vi "longterm_testV2.vi"() -> ()   [LabVIEW 2017]
uses:
  <vilib>/Math Plots/2D Math Plots/2D Error Bar/2D Error Bar XCtrl/2D Error Bar.xctl
  <vilib>/Math Plots/2D Math Plots/2D Error Bar/2D Error Bar Datatype/2D Error Bar Datatype.lvclass
  <vilib>/Math Plots/2D Math Plots/2D Error Bar/2D Error Bar Datatype/Public/Plot Helper (Fixed).vi
panel:
  out "Vcc":T1(graph)=[{"seconds since 1Jan1904"=timestamp(3822506942.315674 s since 1904-01-01), "mean[ps]"=986.572265625}, {"seconds since 1Jan1904"=timestamp(3822507243.6711025 s since 1904-01-01), "mean[ps]"=973.388671875}, {"seconds since 1Jan1904"=timestamp(3822507545.1626496 s since 1904-01-01), "mean[ps]"=984.375}, {"seconds since 1Jan1904"=timestamp(3822507846.553396 s since 1904-01-01), "mean[ps]"=972.65625}, {"seconds since 1Jan1904"=timestamp(3822508148.061275 s since 1904-01-01), "mean[ps]"=972.65625}, {"seconds since 1Jan1904"=timestamp(3822508449.501727 s since 1904-01-01), "mean[ps]"=974.12109375}, {"seconds since 1Jan1904"=timestamp(3822508750.8988624 s since 1904-01-01), "mean[ps]"=974.12109375}, {"seconds since 1Jan1904"=timestamp(3822509052.3161006 s since 1904-01-01), "mean[ps]"=984.375}, {"seconds since 1Jan1904"=timestamp(3822509353.734636 s since 1904-01-01), "mean[ps]"=986.572265625}, {"seconds since 1Jan1904"=timestamp(3822509655.1987686 s since 1904-01-01), "mean[ps]"=972.65625}, {"seconds since 1Jan1904"=timestamp(3822509956.4995074 s since 1904-01-01), "mean[ps]"=974.12109375}, {"seconds since 1Jan1904"=timestamp(3822510257.982245 s since 1904-01-01), "mean[ps]"=984.375}, {"seconds since 1Jan1904"=timestamp(3822510559.3960705 s since 1904-01-01), "mean[ps]"=984.375}, {"seconds since 1Jan1904"=timestamp(3822510860.7242055 s since 1904-01-01), "mean[ps]"=985.83984375}, {"seconds since 1Jan1904"=timestamp(3822511162.215253 s since 1904-01-01), "mean[ps]"=973.388671875}, {"seconds since 1Jan1904"=timestamp(3822511463.639548 s since 1904-01-01), "mean[ps]"=983.642578125}, {"seconds since 1Jan1904"=timestamp(3822511765.766084 s since 1904-01-01), "mean[ps]"=995.361328125}, {"seconds since 1Jan1904"=timestamp(3822512067.2562017 s since 1904-01-01), "mean[ps]"=984.375}, {"seconds since 1Jan1904"=timestamp(3822512368.655607 s since 1904-01-01), "mean[ps]"=995.361328125}, {"seconds since 1Jan1904"=timestamp(3822512670.1464553 s since 1904-01-01), "mean[ps]"=995.361328125}, {"seconds since 1Jan1904"=timestamp(3822512971.507803 s since 1904-01-01), "mean[ps]"=974.12109375}, {"seconds since 1Jan1904"=timestamp(3822513272.925895 s since 1904-01-01), "mean[ps]"=985.107421875}, {"seconds since 1Jan1904"=timestamp(3822513574.303528 s since 1904-01-01), "mean[ps]"=995.361328125}, {"seconds since 1Jan1904"=timestamp(3822513875.706833 s since 1904-01-01), "mean[ps]"=984.375}, {"seconds since 1Jan1904"=timestamp(3822514177.255216 s since 1904-01-01), "mean[ps]"=994.62890625}, {"seconds since 1Jan1904"=timestamp(3822514478.6136312 s since 1904-01-01), "mean[ps]"=984.375}, {"seconds since 1Jan1904"=timestamp(3822514780.1012654 s since 1904-01-01), "mean[ps]"=983.642578125}, {"seconds since 1Jan1904"=timestamp(3822515081.6113095 s since 1904-01-01), "mean[ps]"=985.83984375}, {"seconds since 1Jan1904"=timestamp(3822515382.9461207 s since 1904-01-01), "mean[ps]"=983.642578125}, {"seconds since 1Jan1904"=timestamp(3822515684.3828025 s since 1904-01-01), "mean[ps]"=986.572265625}, {"seconds since 1Jan1904"=timestamp(3822515985.8758097 s since 1904-01-01), "mean[ps]"=995.361328125}, {"seconds since 1Jan1904"=timestamp(3822516287.3353777 s since 1904-01-01), "mean[ps]"=972.65625}, {"seconds since 1Jan1904"=timestamp(3822516588.8038144 s since 1904-01-01), "mean[ps]"=972.65625}, {"seconds since 1Jan1904"=timestamp(3822516890.2282143 s since 1904-01-01), "mean[ps]"=973.388671875}, {"seconds since 1Jan1904"=timestamp(3822517191.6262407 s since 1904-01-01), "mean[ps]"=985.83984375}, {"seconds since 1Jan1904"=timestamp(3822517493.0924606 s since 1904-01-01), "mean[ps]"=972.65625}, {"seconds since 1Jan1904"=timestamp(3822517794.532418 s since 1904-01-01), "mean[ps]"=994.62890625}, {"seconds since 1Jan1904"=timestamp(3822518095.958946 s since 1904-01-01), "mean[ps]"=986.572265625}, {"seconds since 1Jan1904"=timestamp(3822518397.3720393 s since 1904-01-01), "mean[ps]"=994.62890625}, {"seconds since 1Jan1904"=timestamp(3822518698.777503 s since 1904-01-01), "mean[ps]"=987.3046875}, {"seconds since 1Jan1904"=timestamp(3822519000.1937714 s since 1904-01-01), "mean[ps]"=984.375}, {"seconds since 1Jan1904"=timestamp(3822519301.6194086 s since 1904-01-01), "mean[ps]"=974.12109375}, {"seconds since 1Jan1904"=timestamp(3822519603.042124 s since 1904-01-01), "mean[ps]"=973.388671875}, {"seconds since 1Jan1904"=timestamp(3822519904.578883 s since 1904-01-01), "mean[ps]"=984.375}, {"seconds since 1Jan1904"=timestamp(3822520206.0544343 s since 1904-01-01), "mean[ps]"=986.572265625}, {"seconds since 1Jan1904"=timestamp(3822520507.509728 s since 1904-01-01), "mean[ps]"=985.83984375}, {"seconds since 1Jan1904"=timestamp(3822520809.0371656 s since 1904-01-01), "mean[ps]"=976.318359375}, {"seconds since 1Jan1904"=timestamp(3822521110.5518007 s since 1904-01-01), "mean[ps]"=981.4453125}, {"seconds since 1Jan1904"=timestamp(3822521411.9820223 s since 1904-01-01), "mean[ps]"=974.12109375}, {"seconds since 1Jan1904"=timestamp(3822521713.4490914 s since 1904-01-01), "mean[ps]"=972.65625}, {"seconds since 1Jan1904"=timestamp(3822522014.93792 s since 1904-01-01), "mean[ps]"=995.361328125}, {"seconds since 1Jan1904"=timestamp(3822522316.3927464 s since 1904-01-01), "mean[ps]"=984.375}, {"seconds since 1Jan1904"=timestamp(3822522617.8067694 s since 1904-01-01), "mean[ps]"=985.107421875}, {"seconds since 1Jan1904"=timestamp(3822522919.2539024 s since 1904-01-01), "mean[ps]"=984.375}, {"seconds since 1Jan1904"=timestamp(3822523220.6865177 s since 1904-01-01), "mean[ps]"=974.12109375}, {"seconds since 1Jan1904"=timestamp(3822523522.1590304 s since 1904-01-01), "mean[ps]"=985.83984375}, {"seconds since 1Jan1904"=timestamp(3822523823.5384583 s since 1904-01-01), "mean[ps]"=985.107421875}, {"seconds since 1Jan1904"=timestamp(3822524124.9813824 s since 1904-01-01), "mean[ps]"=973.388671875}, {"seconds since 1Jan1904"=timestamp(3822524426.491788 s since 1904-01-01), "mean[ps]"=972.65625}, {"seconds since 1Jan1904"=timestamp(3822524727.9125314 s since 1904-01-01), "mean[ps]"=974.853515625}, {"seconds since 1Jan1904"=timestamp(3822525029.379265 s since 1904-01-01), "mean[ps]"=994.62890625}, {"seconds since 1Jan1904"=timestamp(3822525330.781236 s since 1904-01-01), "mean[ps]"=995.361328125}, {"seconds since 1Jan1904"=timestamp(3822525632.329557 s since 1904-01-01), "mean[ps]"=982.177734375}, {"seconds since 1Jan1904"=timestamp(3822525933.784519 s since 1904-01-01), "mean[ps]"=994.62890625}, {"seconds since 1Jan1904"=timestamp(3822526235.2852225 s since 1904-01-01), "mean[ps]"=974.12109375}, {"seconds since 1Jan1904"=timestamp(3822526536.779774 s since 1904-01-01), "mean[ps]"=985.83984375}, {"seconds since 1Jan1904"=timestamp(3822526838.2156734 s since 1904-01-01), "mean[ps]"=985.107421875}, {"seconds since 1Jan1904"=timestamp(3822527139.721087 s since 1904-01-01), "mean[ps]"=994.62890625}, {"seconds since 1Jan1904"=timestamp(3822527441.1896977 s since 1904-01-01), "mean[ps]"=985.107421875}, {"seconds since 1Jan1904"=timestamp(3822527742.6183696 s since 1904-01-01), "mean[ps]"=972.65625}, {"seconds since 1Jan1904"=timestamp(3822528044.0890102 s since 1904-01-01), "mean[ps]"=985.83984375}, {"seconds since 1Jan1904"=timestamp(3822528345.503568 s since 1904-01-01), "mean[ps]"=985.107421875}, {"seconds since 1Jan1904"=timestamp(3822528646.8947263 s since 1904-01-01), "mean[ps]"=986.572265625}, {"seconds since 1Jan1904"=timestamp(3822528948.387137 s since 1904-01-01), "mean[ps]"=995.361328125}, {"seconds since 1Jan1904"=timestamp(3822529249.822836 s since 1904-01-01), "mean[ps]"=973.388671875}, {"seconds since 1Jan1904"=timestamp(3822529551.2237015 s since 1904-01-01), "mean[ps]"=982.91015625}, {"seconds since 1Jan1904"=timestamp(3822529852.7132487 s since 1904-01-01), "mean[ps]"=972.65625}, {"seconds since 1Jan1904"=timestamp(3822530154.13355 s since 1904-01-01), "mean[ps]"=986.572265625}, {"seconds since 1Jan1904"=timestamp(3822530455.5063615 s since 1904-01-01), "mean[ps]"=973.388671875}, {"seconds since 1Jan1904"=timestamp(3822530756.906737 s since 1904-01-01), "mean[ps]"=972.65625}, {"seconds since 1Jan1904"=timestamp(3822531058.404439 s since 1904-01-01), "mean[ps]"=993.896484375}, {"seconds since 1Jan1904"=timestamp(3822531359.808485 s since 1904-01-01), "mean[ps]"=982.177734375}, {"seconds since 1Jan1904"=timestamp(3822531661.336039 s since 1904-01-01), "mean[ps]"=975.5859375}, {"seconds since 1Jan1904"=timestamp(3822531962.7850113 s since 1904-01-01), "mean[ps]"=984.375}, {"seconds since 1Jan1904"=timestamp(3822532264.2264094 s since 1904-01-01), "mean[ps]"=973.388671875}, {"seconds since 1Jan1904"=timestamp(3822532565.644325 s since 1904-01-01), "mean[ps]"=973.388671875}, {"seconds since 1Jan1904"=timestamp(3822532867.095218 s since 1904-01-01), "mean[ps]"=987.3046875}, {"seconds since 1Jan1904"=timestamp(3822533168.4954033 s since 1904-01-01), "mean[ps]"=982.91015625}, {"seconds since 1Jan1904"=timestamp(3822533470.0292826 s since 1904-01-01), "mean[ps]"=984.375}, {"seconds since 1Jan1904"=timestamp(3822533771.460639 s since 1904-01-01), "mean[ps]"=974.12109375}, {"seconds since 1Jan1904"=timestamp(3822534072.903432 s since 1904-01-01), "mean[ps]"=984.375}, {"seconds since 1Jan1904"=timestamp(3822534374.327941 s since 1904-01-01), "mean[ps]"=985.107421875}, {"seconds since 1Jan1904"=timestamp(3822534675.8510175 s since 1904-01-01), "mean[ps]"=983.642578125}, {"seconds since 1Jan1904"=timestamp(3822534977.3926754 s since 1904-01-01), "mean[ps]"=975.5859375}, {"seconds since 1Jan1904"=timestamp(3822535278.8113256 s since 1904-01-01), "mean[ps]"=985.83984375}, {"seconds since 1Jan1904"=timestamp(3822535580.052392 s since 1904-01-01), "mean[ps]"=973.388671875}, {"seconds since 1Jan1904"=timestamp(3822535881.6109457 s since 1904-01-01), "mean[ps]"=993.1640625}, {"seconds since 1Jan1904"=timestamp(3822536183.1016607 s since 1904-01-01), "mean[ps]"=987.3046875}, {"seconds since 1Jan1904"=timestamp(3822536484.4703193 s since 1904-01-01), "mean[ps]"=994.62890625}, {"seconds since 1Jan1904"=timestamp(3822536786.003652 s since 1904-01-01), "mean[ps]"=993.896484375}, {"seconds since 1Jan1904"=timestamp(3822537087.3877025 s since 1904-01-01), "mean[ps]"=995.361328125}, {"seconds since 1Jan1904"=timestamp(3822537388.9627695 s since 1904-01-01), "mean[ps]"=974.853515625}, {"seconds since 1Jan1904"=timestamp(3822537690.32478 s since 1904-01-01), "mean[ps]"=993.896484375}, {"seconds since 1Jan1904"=timestamp(3822537991.8736057 s since 1904-01-01), "mean[ps]"=994.62890625}, {"seconds since 1Jan1904"=timestamp(3822538293.281887 s since 1904-01-01), "mean[ps]"=972.65625}, {"seconds since 1Jan1904"=timestamp(3822538594.700456 s since 1904-01-01), "mean[ps]"=972.65625}, {"seconds since 1Jan1904"=timestamp(3822538896.2253175 s since 1904-01-01), "mean[ps]"=972.65625}, {"seconds since 1Jan1904"=timestamp(3822539197.7020054 s since 1904-01-01), "mean[ps]"=985.83984375}, {"seconds since 1Jan1904"=timestamp(3822539499.1529503 s since 1904-01-01), "mean[ps]"=995.361328125}, {"seconds since 1Jan1904"=timestamp(3822539800.5176826 s since 1904-01-01), "mean[ps]"=983.642578125}, {"seconds since 1Jan1904"=timestamp(3822540101.955672 s since 1904-01-01), "mean[ps]"=972.65625}, {"seconds since 1Jan1904"=timestamp(3822540403.389026 s since 1904-01-01), "mean[ps]"=985.83984375}, {"seconds since 1Jan1904"=timestamp(3822540704.8647823 s since 1904-01-01), "mean[ps]"=986.572265625}, {"seconds since 1Jan1904"=timestamp(3822541006.2905207 s since 1904-01-01), "mean[ps]"=985.83984375}, {"seconds since 1Jan1904"=timestamp(3822541307.8066297 s since 1904-01-01), "mean[ps]"=986.572265625}, {"seconds since 1Jan1904"=timestamp(3822541609.3079934 s since 1904-01-01), "mean[ps]"=972.65625}, {"seconds since 1Jan1904"=timestamp(3822541910.788964 s since 1904-01-01), "mean[ps]"=985.107421875}, {"seconds since 1Jan1904"=timestamp(3822542212.360313 s since 1904-01-01), "mean[ps]"=984.375}, {"seconds since 1Jan1904"=timestamp(3822542513.8452806 s since 1904-01-01), "mean[ps]"=984.375}, {"seconds since 1Jan1904"=timestamp(3822542815.328869 s since 1904-01-01), "mean[ps]"=972.65625}, {"seconds since 1Jan1904"=timestamp(3822543116.8031616 s since 1904-01-01), "mean[ps]"=982.91015625}, {"seconds since 1Jan1904"=timestamp(3822543418.253579 s since 1904-01-01), "mean[ps]"=985.83984375}, {"seconds since 1Jan1904"=timestamp(3822543719.8005633 s since 1904-01-01), "mean[ps]"=982.91015625}, {"seconds since 1Jan1904"=timestamp(3822544021.284577 s since 1904-01-01), "mean[ps]"=982.177734375}, {"seconds since 1Jan1904"=timestamp(3822544322.8030105 s since 1904-01-01), "mean[ps]"=986.572265625}, {"seconds since 1Jan1904"=timestamp(3822544624.2975945 s since 1904-01-01), "mean[ps]"=984.375}, {"seconds since 1Jan1904"=timestamp(3822544925.818383 s since 1904-01-01), "mean[ps]"=985.107421875}, {"seconds since 1Jan1904"=timestamp(3822545227.2305446 s since 1904-01-01), "mean[ps]"=983.642578125}, {"seconds since 1Jan1904"=timestamp(3822545528.6374345 s since 1904-01-01), "mean[ps]"=995.361328125}, {"seconds since 1Jan1904"=timestamp(3822545830.161919 s since 1904-01-01), "mean[ps]"=972.65625}, {"seconds since 1Jan1904"=timestamp(3822546131.6581616 s since 1904-01-01), "mean[ps]"=985.107421875}, {"seconds since 1Jan1904"=timestamp(3822546433.1208367 s since 1904-01-01), "mean[ps]"=973.388671875}, {"seconds since 1Jan1904"=timestamp(3822546734.5235424 s since 1904-01-01), "mean[ps]"=984.375}, {"seconds since 1Jan1904"=timestamp(3822547035.9215217 s since 1904-01-01), "mean[ps]"=972.65625}, {"seconds since 1Jan1904"=timestamp(3822547337.4649706 s since 1904-01-01), "mean[ps]"=972.65625}, {"seconds since 1Jan1904"=timestamp(3822547638.88064 s since 1904-01-01), "mean[ps]"=982.91015625}, {"seconds since 1Jan1904"=timestamp(3822547940.3121905 s since 1904-01-01), "mean[ps]"=973.388671875}, {"seconds since 1Jan1904"=timestamp(3822548241.74978 s since 1904-01-01), "mean[ps]"=984.375}, {"seconds since 1Jan1904"=timestamp(3822548543.2799606 s since 1904-01-01), "mean[ps]"=973.388671875}, {"seconds since 1Jan1904"=timestamp(3822548844.742632 s since 1904-01-01), "mean[ps]"=985.107421875}, {"seconds since 1Jan1904"=timestamp(3822549146.149104 s since 1904-01-01), "mean[ps]"=984.375}, {"seconds since 1Jan1904"=timestamp(3822549447.533661 s since 1904-01-01), "mean[ps]"=985.107421875}, {"seconds since 1Jan1904"=timestamp(3822549748.9579425 s since 1904-01-01), "mean[ps]"=995.361328125}, {"seconds since 1Jan1904"=timestamp(3822550050.4716654 s since 1904-01-01), "mean[ps]"=985.83984375}, {"seconds since 1Jan1904"=timestamp(3822550351.947339 s since 1904-01-01), "mean[ps]"=985.107421875}, {"seconds since 1Jan1904"=timestamp(3822550653.458123 s since 1904-01-01), "mean[ps]"=983.642578125}, {"seconds since 1Jan1904"=timestamp(3822550954.99518 s since 1904-01-01), "mean[ps]"=985.83984375}, {"seconds since 1Jan1904"=timestamp(3822551256.5036974 s since 1904-01-01), "mean[ps]"=985.107421875}, {"seconds since 1Jan1904"=timestamp(3822551558.0137887 s since 1904-01-01), "mean[ps]"=995.361328125}, {"seconds since 1Jan1904"=timestamp(3822551859.5051265 s since 1904-01-01), "mean[ps]"=995.361328125}, {"seconds since 1Jan1904"=timestamp(3822552161.039615 s since 1904-01-01), "mean[ps]"=986.572265625}, {"seconds since 1Jan1904"=timestamp(3822552462.609901 s since 1904-01-01), "mean[ps]"=974.853515625}, {"seconds since 1Jan1904"=timestamp(3822552764.000548 s since 1904-01-01), "mean[ps]"=985.107421875}, {"seconds since 1Jan1904"=timestamp(3822553065.419496 s since 1904-01-01), "mean[ps]"=984.375}, {"seconds since 1Jan1904"=timestamp(3822553366.9214015 s since 1904-01-01), "mean[ps]"=995.361328125}, {"seconds since 1Jan1904"=timestamp(3822553668.2656054 s since 1904-01-01), "mean[ps]"=984.375}, {"seconds since 1Jan1904"=timestamp(3822553969.7844114 s since 1904-01-01), "mean[ps]"=984.375}, {"seconds since 1Jan1904"=timestamp(3822554271.2343993 s since 1904-01-01), "mean[ps]"=984.375}, {"seconds since 1Jan1904"=timestamp(3822554572.7825623 s since 1904-01-01), "mean[ps]"=983.642578125}, {"seconds since 1Jan1904"=timestamp(3822554874.2372446 s since 1904-01-01), "mean[ps]"=984.375}, {"seconds since 1Jan1904"=timestamp(3822555175.792369 s since 1904-01-01), "mean[ps]"=985.107421875}, {"seconds since 1Jan1904"=timestamp(3822555477.2372074 s since 1904-01-01), "mean[ps]"=972.65625}, {"seconds since 1Jan1904"=timestamp(3822555778.701035 s since 1904-01-01), "mean[ps]"=987.3046875}, {"seconds since 1Jan1904"=timestamp(3822556080.2516418 s since 1904-01-01), "mean[ps]"=974.12109375}, {"seconds since 1Jan1904"=timestamp(3822556381.757804 s since 1904-01-01), "mean[ps]"=985.107421875}, {"seconds since 1Jan1904"=timestamp(3822556683.148675 s since 1904-01-01), "mean[ps]"=972.65625}, {"seconds since 1Jan1904"=timestamp(3822556984.6444607 s since 1904-01-01), "mean[ps]"=985.107421875}, {"seconds since 1Jan1904"=timestamp(3822557286.095585 s since 1904-01-01), "mean[ps]"=982.91015625}, {"seconds since 1Jan1904"=timestamp(3822557587.5588975 s since 1904-01-01), "mean[ps]"=985.83984375}, {"seconds since 1Jan1904"=timestamp(3822557889.0395904 s since 1904-01-01), "mean[ps]"=974.853515625}, {"seconds since 1Jan1904"=timestamp(3822558190.4474607 s since 1904-01-01), "mean[ps]"=985.107421875}, {"seconds since 1Jan1904"=timestamp(3822558492.0190606 s since 1904-01-01), "mean[ps]"=983.642578125}, {"seconds since 1Jan1904"=timestamp(3822558793.477814 s since 1904-01-01), "mean[ps]"=985.83984375}, {"seconds since 1Jan1904"=timestamp(3822559094.921321 s since 1904-01-01), "mean[ps]"=994.62890625}, {"seconds since 1Jan1904"=timestamp(3822559396.4460673 s since 1904-01-01), "mean[ps]"=984.375}, {"seconds since 1Jan1904"=timestamp(3822559697.9183455 s since 1904-01-01), "mean[ps]"=973.388671875}, {"seconds since 1Jan1904"=timestamp(3822559999.3983808 s since 1904-01-01), "mean[ps]"=994.62890625}, {"seconds since 1Jan1904"=timestamp(3822560300.8987856 s since 1904-01-01), "mean[ps]"=974.12109375}, {"seconds since 1Jan1904"=timestamp(3822560602.3556256 s since 1904-01-01), "mean[ps]"=974.853515625}, {"seconds since 1Jan1904"=timestamp(3822560903.899011 s since 1904-01-01), "mean[ps]"=981.4453125}, {"seconds since 1Jan1904"=timestamp(3822561205.442392 s since 1904-01-01), "mean[ps]"=994.62890625}, {"seconds since 1Jan1904"=timestamp(3822561506.864459 s since 1904-01-01), "mean[ps]"=986.572265625}, {"seconds since 1Jan1904"=timestamp(3822561808.4265895 s since 1904-01-01), "mean[ps]"=985.107421875}, {"seconds since 1Jan1904"=timestamp(3822562109.9678545 s since 1904-01-01), "mean[ps]"=972.65625}, {"seconds since 1Jan1904"=timestamp(3822562411.5341334 s since 1904-01-01), "mean[ps]"=982.91015625}, {"seconds since 1Jan1904"=timestamp(3822562712.998142 s since 1904-01-01), "mean[ps]"=994.62890625}, {"seconds since 1Jan1904"=timestamp(3822563014.480204 s since 1904-01-01), "mean[ps]"=995.361328125}, {"seconds since 1Jan1904"=timestamp(3822563315.9980226 s since 1904-01-01), "mean[ps]"=973.388671875}, {"seconds since 1Jan1904"=timestamp(3822563617.240683 s since 1904-01-01), "mean[ps]"=972.65625}, {"seconds since 1Jan1904"=timestamp(3822563918.749057 s since 1904-01-01), "mean[ps]"=984.375}, {"seconds since 1Jan1904"=timestamp(3822564220.254855 s since 1904-01-01), "mean[ps]"=985.107421875}, {"seconds since 1Jan1904"=timestamp(3822564521.8313217 s since 1904-01-01), "mean[ps]"=985.83984375}, {"seconds since 1Jan1904"=timestamp(3822564823.2753153 s since 1904-01-01), "mean[ps]"=985.107421875}, {"seconds since 1Jan1904"=timestamp(3822565124.701639 s since 1904-01-01), "mean[ps]"=985.83984375}, {"seconds since 1Jan1904"=timestamp(3822565426.1726537 s since 1904-01-01), "mean[ps]"=986.572265625}, {"seconds since 1Jan1904"=timestamp(3822565727.6830926 s since 1904-01-01), "mean[ps]"=972.65625}, {"seconds since 1Jan1904"=timestamp(3822566029.165819 s since 1904-01-01), "mean[ps]"=974.12109375}, {"seconds since 1Jan1904"=timestamp(3822566330.740963 s since 1904-01-01), "mean[ps]"=972.65625}, {"seconds since 1Jan1904"=timestamp(3822566632.249509 s since 1904-01-01), "mean[ps]"=983.642578125}, {"seconds since 1Jan1904"=timestamp(3822566933.704676 s since 1904-01-01), "mean[ps]"=972.65625}, {"seconds since 1Jan1904"=timestamp(3822567235.209213 s since 1904-01-01), "mean[ps]"=984.375}, {"seconds since 1Jan1904"=timestamp(3822567536.6946225 s since 1904-01-01), "mean[ps]"=994.62890625}, {"seconds since 1Jan1904"=timestamp(3822567838.169631 s since 1904-01-01), "mean[ps]"=982.91015625}, {"seconds since 1Jan1904"=timestamp(3822568139.6286063 s since 1904-01-01), "mean[ps]"=985.83984375}, {"seconds since 1Jan1904"=timestamp(3822568441.096488 s since 1904-01-01), "mean[ps]"=995.361328125}, {"seconds since 1Jan1904"=timestamp(3822568742.5332594 s since 1904-01-01), "mean[ps]"=984.375}, {"seconds since 1Jan1904"=timestamp(3822569044.0896015 s since 1904-01-01), "mean[ps]"=972.65625}, {"seconds since 1Jan1904"=timestamp(3822569345.551961 s since 1904-01-01), "mean[ps]"=987.3046875}, {"seconds since 1Jan1904"=timestamp(3822569647.024821 s since 1904-01-01), "mean[ps]"=994.62890625}, {"seconds since 1Jan1904"=timestamp(3822569948.559713 s since 1904-01-01), "mean[ps]"=986.572265625}, {"seconds since 1Jan1904"=timestamp(3822570249.9499383 s since 1904-01-01), "mean[ps]"=995.361328125}, {"seconds since 1Jan1904"=timestamp(3822570551.4543366 s since 1904-01-01), "mean[ps]"=974.12109375}, {"seconds since 1Jan1904"=timestamp(3822570852.907388 s since 1904-01-01), "mean[ps]"=985.107421875}, {"seconds since 1Jan1904"=timestamp(3822571154.3613434 s since 1904-01-01), "mean[ps]"=973.388671875}, {"seconds since 1Jan1904"=timestamp(3822571455.875889 s since 1904-01-01), "mean[ps]"=975.5859375}, {"seconds since 1Jan1904"=timestamp(3822571757.4035335 s since 1904-01-01), "mean[ps]"=984.375}, {"seconds since 1Jan1904"=timestamp(3822572058.8738127 s since 1904-01-01), "mean[ps]"=983.642578125}, {"seconds since 1Jan1904"=timestamp(3822572360.3478255 s since 1904-01-01), "mean[ps]"=995.361328125}, {"seconds since 1Jan1904"=timestamp(3822572661.834789 s since 1904-01-01), "mean[ps]"=985.107421875}, {"seconds since 1Jan1904"=timestamp(3822572963.3136296 s since 1904-01-01), "mean[ps]"=983.642578125}, {"seconds since 1Jan1904"=timestamp(3822573264.8089194 s since 1904-01-01), "mean[ps]"=987.3046875}, {"seconds since 1Jan1904"=timestamp(3822573566.2905793 s since 1904-01-01), "mean[ps]"=983.642578125}, {"seconds since 1Jan1904"=timestamp(3822573867.753861 s since 1904-01-01), "mean[ps]"=982.91015625}, {"seconds since 1Jan1904"=timestamp(3822574169.3307586 s since 1904-01-01), "mean[ps]"=985.83984375}, {"seconds since 1Jan1904"=timestamp(3822574470.7852354 s since 1904-01-01), "mean[ps]"=988.037109375}, {"seconds since 1Jan1904"=timestamp(3822574772.1922865 s since 1904-01-01), "mean[ps]"=984.375}, {"seconds since 1Jan1904"=timestamp(3822575073.6485744 s since 1904-01-01), "mean[ps]"=982.91015625}, {"seconds since 1Jan1904"=timestamp(3822575375.0628457 s since 1904-01-01), "mean[ps]"=994.62890625}, {"seconds since 1Jan1904"=timestamp(3822575676.540885 s since 1904-01-01), "mean[ps]"=984.375}, {"seconds since 1Jan1904"=timestamp(3822575978.110875 s since 1904-01-01), "mean[ps]"=972.65625}, {"seconds since 1Jan1904"=timestamp(3822576279.6679864 s since 1904-01-01), "mean[ps]"=982.91015625}, {"seconds since 1Jan1904"=timestamp(3822576581.2032743 s since 1904-01-01), "mean[ps]"=984.375}, {"seconds since 1Jan1904"=timestamp(3822576882.6405673 s since 1904-01-01), "mean[ps]"=985.83984375}, {"seconds since 1Jan1904"=timestamp(3822577184.1204553 s since 1904-01-01), "mean[ps]"=994.62890625}, {"seconds since 1Jan1904"=timestamp(3822577485.6404696 s since 1904-01-01), "mean[ps]"=973.388671875}, {"seconds since 1Jan1904"=timestamp(3822577787.095057 s since 1904-01-01), "mean[ps]"=982.91015625}, {"seconds since 1Jan1904"=timestamp(3822578088.553026 s since 1904-01-01), "mean[ps]"=984.375}, {"seconds since 1Jan1904"=timestamp(3822578390.115008 s since 1904-01-01), "mean[ps]"=982.91015625}, {"seconds since 1Jan1904"=timestamp(3822578691.551293 s since 1904-01-01), "mean[ps]"=995.361328125}, {"seconds since 1Jan1904"=timestamp(3822578992.9199705 s since 1904-01-01), "mean[ps]"=994.62890625}, {"seconds since 1Jan1904"=timestamp(3822579294.3933854 s since 1904-01-01), "mean[ps]"=995.361328125}, {"seconds since 1Jan1904"=timestamp(3822579595.918991 s since 1904-01-01), "mean[ps]"=995.361328125}, {"seconds since 1Jan1904"=timestamp(3822579897.4222097 s since 1904-01-01), "mean[ps]"=982.177734375}, {"seconds since 1Jan1904"=timestamp(3822580198.9128265 s since 1904-01-01), "mean[ps]"=975.5859375}, {"seconds since 1Jan1904"=timestamp(3822580500.314174 s since 1904-01-01), "mean[ps]"=986.572265625}, {"seconds since 1Jan1904"=timestamp(3822580801.8501215 s since 1904-01-01), "mean[ps]"=988.037109375}, {"seconds since 1Jan1904"=timestamp(3822581103.3778 s since 1904-01-01), "mean[ps]"=973.388671875}, {"seconds since 1Jan1904"=timestamp(3822581404.880745 s since 1904-01-01), "mean[ps]"=983.642578125}, {"seconds since 1Jan1904"=timestamp(3822581706.4360175 s since 1904-01-01), "mean[ps]"=984.375}, {"seconds since 1Jan1904"=timestamp(3822582007.8203206 s since 1904-01-01), "mean[ps]"=995.361328125}, {"seconds since 1Jan1904"=timestamp(3822582309.2484713 s since 1904-01-01), "mean[ps]"=995.361328125}, {"seconds since 1Jan1904"=timestamp(3822582610.7182074 s since 1904-01-01), "mean[ps]"=974.12109375}, {"seconds since 1Jan1904"=timestamp(3822582912.221481 s since 1904-01-01), "mean[ps]"=980.712890625}, {"seconds since 1Jan1904"=timestamp(3822583213.701206 s since 1904-01-01), "mean[ps]"=973.388671875}, {"seconds since 1Jan1904"=timestamp(3822583515.2400217 s since 1904-01-01), "mean[ps]"=982.177734375}, {"seconds since 1Jan1904"=timestamp(3822583816.7411456 s since 1904-01-01), "mean[ps]"=982.91015625}, {"seconds since 1Jan1904"=timestamp(3822584118.2147617 s since 1904-01-01), "mean[ps]"=982.91015625}, {"seconds since 1Jan1904"=timestamp(3822584419.675927 s since 1904-01-01), "mean[ps]"=995.361328125}, {"seconds since 1Jan1904"=timestamp(3822584721.0923023 s since 1904-01-01), "mean[ps]"=986.572265625}, {"seconds since 1Jan1904"=timestamp(3822585022.5496383 s since 1904-01-01), "mean[ps]"=976.318359375}, {"seconds since 1Jan1904"=timestamp(3822585324.043527 s since 1904-01-01), "mean[ps]"=974.853515625}, {"seconds since 1Jan1904"=timestamp(3822585625.471996 s since 1904-01-01), "mean[ps]"=972.65625}, {"seconds since 1Jan1904"=timestamp(3822585926.8942423 s since 1904-01-01), "mean[ps]"=975.5859375}, {"seconds since 1Jan1904"=timestamp(3822586228.3225694 s since 1904-01-01), "mean[ps]"=986.572265625}, {"seconds since 1Jan1904"=timestamp(3822586529.8338766 s since 1904-01-01), "mean[ps]"=986.572265625}, {"seconds since 1Jan1904"=timestamp(3822586831.2920294 s since 1904-01-01), "mean[ps]"=986.572265625}, {"seconds since 1Jan1904"=timestamp(3822587132.7088814 s since 1904-01-01), "mean[ps]"=985.107421875}, {"seconds since 1Jan1904"=timestamp(3822587434.1071906 s since 1904-01-01), "mean[ps]"=986.572265625}, {"seconds since 1Jan1904"=timestamp(3822587735.3207207 s since 1904-01-01), "mean[ps]"=986.572265625}, {"seconds since 1Jan1904"=timestamp(3822588036.7855854 s since 1904-01-01), "mean[ps]"=985.107421875}, {"seconds since 1Jan1904"=timestamp(3822588338.3446593 s since 1904-01-01), "mean[ps]"=982.91015625}, {"seconds since 1Jan1904"=timestamp(3822588639.839839 s since 1904-01-01), "mean[ps]"=992.431640625}, {"seconds since 1Jan1904"=timestamp(3822588941.288984 s since 1904-01-01), "mean[ps]"=985.83984375}, {"seconds since 1Jan1904"=timestamp(3822589242.7402463 s since 1904-01-01), "mean[ps]"=995.361328125}, {"seconds since 1Jan1904"=timestamp(3822589544.2098656 s since 1904-01-01), "mean[ps]"=983.642578125}, {"seconds since 1Jan1904"=timestamp(3822589845.6971216 s since 1904-01-01), "mean[ps]"=973.388671875}, {"seconds since 1Jan1904"=timestamp(3822590147.2125216 s since 1904-01-01), "mean[ps]"=982.91015625}, {"seconds since 1Jan1904"=timestamp(3822590448.640258 s since 1904-01-01), "mean[ps]"=972.65625}, {"seconds since 1Jan1904"=timestamp(3822590750.1391034 s since 1904-01-01), "mean[ps]"=993.896484375}, {"seconds since 1Jan1904"=timestamp(3822591051.5836415 s since 1904-01-01), "mean[ps]"=976.318359375}, {"seconds since 1Jan1904"=timestamp(3822591352.9831247 s since 1904-01-01), "mean[ps]"=973.388671875}, {"seconds since 1Jan1904"=timestamp(3822591654.485979 s since 1904-01-01), "mean[ps]"=986.572265625}, {"seconds since 1Jan1904"=timestamp(3822591955.859042 s since 1904-01-01), "mean[ps]"=995.361328125}, {"seconds since 1Jan1904"=timestamp(3822592257.408669 s since 1904-01-01), "mean[ps]"=972.65625}, {"seconds since 1Jan1904"=timestamp(3822592558.932187 s since 1904-01-01), "mean[ps]"=984.375}, {"seconds since 1Jan1904"=timestamp(3822592860.391513 s since 1904-01-01), "mean[ps]"=993.896484375}, {"seconds since 1Jan1904"=timestamp(3822593161.860652 s since 1904-01-01), "mean[ps]"=983.642578125}, {"seconds since 1Jan1904"=timestamp(3822593463.385323 s since 1904-01-01), "mean[ps]"=985.107421875}, {"seconds since 1Jan1904"=timestamp(3822593764.8500686 s since 1904-01-01), "mean[ps]"=985.83984375}, {"seconds since 1Jan1904"=timestamp(3822594066.308588 s since 1904-01-01), "mean[ps]"=981.4453125}, {"seconds since 1Jan1904"=timestamp(3822594367.780607 s since 1904-01-01), "mean[ps]"=985.83984375}, {"seconds since 1Jan1904"=timestamp(3822594669.2577024 s since 1904-01-01), "mean[ps]"=982.91015625}, {"seconds since 1Jan1904"=timestamp(3822594970.726291 s since 1904-01-01), "mean[ps]"=985.83984375}, {"seconds since 1Jan1904"=timestamp(3822595272.1390114 s since 1904-01-01), "mean[ps]"=973.388671875}, {"seconds since 1Jan1904"=timestamp(3822595573.6779704 s since 1904-01-01), "mean[ps]"=994.62890625}, {"seconds since 1Jan1904"=timestamp(3822595875.2007656 s since 1904-01-01), "mean[ps]"=984.375}, {"seconds since 1Jan1904"=timestamp(3822596176.6578298 s since 1904-01-01), "mean[ps]"=985.107421875}, {"seconds since 1Jan1904"=timestamp(3822596478.2190976 s since 1904-01-01), "mean[ps]"=974.12109375}, {"seconds since 1Jan1904"=timestamp(3822596779.7422447 s since 1904-01-01), "mean[ps]"=985.107421875}, {"seconds since 1Jan1904"=timestamp(3822597081.1809144 s since 1904-01-01), "mean[ps]"=985.83984375}, {"seconds since 1Jan1904"=timestamp(3822597382.686327 s since 1904-01-01), "mean[ps]"=985.83984375}, {"seconds since 1Jan1904"=timestamp(3822597684.2478952 s since 1904-01-01), "mean[ps]"=984.375}, {"seconds since 1Jan1904"=timestamp(3822597985.7226458 s since 1904-01-01), "mean[ps]"=984.375}, {"seconds since 1Jan1904"=timestamp(3822598287.212348 s since 1904-01-01), "mean[ps]"=995.361328125}, {"seconds since 1Jan1904"=timestamp(3822598588.6026154 s since 1904-01-01), "mean[ps]"=993.896484375}, {"seconds since 1Jan1904"=timestamp(3822598890.0572553 s since 1904-01-01), "mean[ps]"=987.3046875}, {"seconds since 1Jan1904"=timestamp(3822599191.425584 s since 1904-01-01), "mean[ps]"=973.388671875}, {"seconds since 1Jan1904"=timestamp(3822599492.866769 s since 1904-01-01), "mean[ps]"=985.107421875}, {"seconds since 1Jan1904"=timestamp(3822599794.2904983 s since 1904-01-01), "mean[ps]"=973.388671875}, {"seconds since 1Jan1904"=timestamp(3822600095.7871695 s since 1904-01-01), "mean[ps]"=973.388671875}, {"seconds since 1Jan1904"=timestamp(3822600397.4508214 s since 1904-01-01), "mean[ps]"=983.642578125}, {"seconds since 1Jan1904"=timestamp(3822600698.83722 s since 1904-01-01), "mean[ps]"=994.62890625}, {"seconds since 1Jan1904"=timestamp(3822601000.21038 s since 1904-01-01), "mean[ps]"=973.388671875}, {"seconds since 1Jan1904"=timestamp(3822601301.7260976 s since 1904-01-01), "mean[ps]"=973.388671875}]
  in  "mean[ps] 4":dbl=-0.9 format="%0.2f"
  in  "mean[ps] 3":dbl=-0.7 format="%0.2f"
  in  "seconds since 1Jan1904 3":timestamp=timestamp(3822019516.105 s since 1904-01-01)
  in  "mean[ps] 2":dbl=-0.16666666666666666 format="%0.2f"
  in  "seconds since 1Jan1904 2":timestamp=timestamp(3822019276.105 s since 1904-01-01)
  out "Mean 2":T2(graph)=[{[{"seconds since 1Jan1904 2"=timestamp(3822019276.105 s since 1904-01-01), "mean[ps] 2"=-0.16666666666666666}, {"seconds since 1Jan1904 2"=timestamp(3822019516.105 s since 1904-01-01), "mean[ps] 2"=-0.7}]}, {[{"seconds since 1Jan1904 2"=timestamp(3822019276.105 s since 1904-01-01), "mean[ps] 2"=-0.16666666666666666}, {"seconds since 1Jan1904 2"=timestamp(3822019516.105 s since 1904-01-01), "mean[ps] 2"=-0.9}]}]
  out "temperature":T1(graph)=[{"seconds since 1Jan1904"=timestamp(3822506942.315674 s since 1904-01-01), "mean[ps]"=40.85004882812501}, {"seconds since 1Jan1904"=timestamp(3822507243.6711025 s since 1904-01-01), "mean[ps]"=41.465252685546886}, {"seconds since 1Jan1904"=timestamp(3822507545.1626496 s since 1904-01-01), "mean[ps]"=41.465252685546886}, {"seconds since 1Jan1904"=timestamp(3822507846.553396 s since 1904-01-01), "mean[ps]"=40.97308959960941}, {"seconds since 1Jan1904"=timestamp(3822508148.061275 s since 1904-01-01), "mean[ps]"=41.588293457031284}, {"seconds since 1Jan1904"=timestamp(3822508449.501727 s since 1904-01-01), "mean[ps]"=41.342211914062545}, {"seconds since 1Jan1904"=timestamp(3822508750.8988624 s since 1904-01-01), "mean[ps]"=72.47152709960943}, {"seconds since 1Jan1904"=timestamp(3822509052.3161006 s since 1904-01-01), "mean[ps]"=10.335937500000057}, {"seconds since 1Jan1904"=timestamp(3822509353.734636 s since 1904-01-01), "mean[ps]"=41.342211914062545}, {"seconds since 1Jan1904"=timestamp(3822509655.1987686 s since 1904-01-01), "mean[ps]"=40.85004882812501}, {"seconds since 1Jan1904"=timestamp(3822509956.4995074 s since 1904-01-01), "mean[ps]"=41.588293457031284}, {"seconds since 1Jan1904"=timestamp(3822510257.982245 s since 1904-01-01), "mean[ps]"=72.96369018554691}, {"seconds since 1Jan1904"=timestamp(3822510559.3960705 s since 1904-01-01), "mean[ps]"=41.09613037109381}, {"seconds since 1Jan1904"=timestamp(3822510860.7242055 s since 1904-01-01), "mean[ps]"=40.85004882812501}, {"seconds since 1Jan1904"=timestamp(3822511162.215253 s since 1904-01-01), "mean[ps]"=41.21917114257815}, {"seconds since 1Jan1904"=timestamp(3822511463.639548 s since 1904-01-01), "mean[ps]"=42.32653808593756}, {"seconds since 1Jan1904"=timestamp(3822511765.766084 s since 1904-01-01), "mean[ps]"=41.83437500000002}, {"seconds since 1Jan1904"=timestamp(3822512067.2562017 s since 1904-01-01), "mean[ps]"=41.588293457031284}, {"seconds since 1Jan1904"=timestamp(3822512368.655607 s since 1904-01-01), "mean[ps]"=42.32653808593756}, {"seconds since 1Jan1904"=timestamp(3822512670.1464553 s since 1904-01-01), "mean[ps]"=41.71133422851568}, {"seconds since 1Jan1904"=timestamp(3822512971.507803 s since 1904-01-01), "mean[ps]"=10.335937500000057}, {"seconds since 1Jan1904"=timestamp(3822513272.925895 s since 1904-01-01), "mean[ps]"=10.458978271484398}, {"seconds since 1Jan1904"=timestamp(3822513574.303528 s since 1904-01-01), "mean[ps]"=42.20349731445316}, {"seconds since 1Jan1904"=timestamp(3822513875.706833 s since 1904-01-01), "mean[ps]"=73.0867309570313}, {"seconds since 1Jan1904"=timestamp(3822514177.255216 s since 1904-01-01), "mean[ps]"=42.08045654296876}, {"seconds since 1Jan1904"=timestamp(3822514478.6136312 s since 1904-01-01), "mean[ps]"=72.96369018554691}, {"seconds since 1Jan1904"=timestamp(3822514780.1012654 s since 1904-01-01), "mean[ps]"=10.828100585937534}, {"seconds since 1Jan1904"=timestamp(3822515081.6113095 s since 1904-01-01), "mean[ps]"=11.074182128906273}, {"seconds since 1Jan1904"=timestamp(3822515382.9461207 s since 1904-01-01), "mean[ps]"=72.59456787109377}, {"seconds since 1Jan1904"=timestamp(3822515684.3828025 s since 1904-01-01), "mean[ps]"=41.83437500000002}, {"seconds since 1Jan1904"=timestamp(3822515985.8758097 s since 1904-01-01), "mean[ps]"=42.32653808593756}, {"seconds since 1Jan1904"=timestamp(3822516287.3353777 s since 1904-01-01), "mean[ps]"=42.32653808593756}, {"seconds since 1Jan1904"=timestamp(3822516588.8038144 s since 1904-01-01), "mean[ps]"=42.20349731445316}, {"seconds since 1Jan1904"=timestamp(3822516890.2282143 s since 1904-01-01), "mean[ps]"=42.818701171875034}, {"seconds since 1Jan1904"=timestamp(3822517191.6262407 s since 1904-01-01), "mean[ps]"=42.695660400390636}, {"seconds since 1Jan1904"=timestamp(3822517493.0924606 s since 1904-01-01), "mean[ps]"=42.4495788574219}, {"seconds since 1Jan1904"=timestamp(3822517794.532418 s since 1904-01-01), "mean[ps]"=41.95741577148442}, {"seconds since 1Jan1904"=timestamp(3822518095.958946 s since 1904-01-01), "mean[ps]"=43.18782348632817}, {"seconds since 1Jan1904"=timestamp(3822518397.3720393 s since 1904-01-01), "mean[ps]"=42.572619628906295}, {"seconds since 1Jan1904"=timestamp(3822518698.777503 s since 1904-01-01), "mean[ps]"=43.06478271484377}, {"seconds since 1Jan1904"=timestamp(3822519000.1937714 s since 1904-01-01), "mean[ps]"=42.4495788574219}, {"seconds since 1Jan1904"=timestamp(3822519301.6194086 s since 1904-01-01), "mean[ps]"=42.4495788574219}, {"seconds since 1Jan1904"=timestamp(3822519603.042124 s since 1904-01-01), "mean[ps]"=42.695660400390636}, {"seconds since 1Jan1904"=timestamp(3822519904.578883 s since 1904-01-01), "mean[ps]"=42.94174194335943}, {"seconds since 1Jan1904"=timestamp(3822520206.0544343 s since 1904-01-01), "mean[ps]"=42.695660400390636}, {"seconds since 1Jan1904"=timestamp(3822520507.509728 s since 1904-01-01), "mean[ps]"=42.08045654296876}, {"seconds since 1Jan1904"=timestamp(3822520809.0371656 s since 1904-01-01), "mean[ps]"=43.06478271484377}, {"seconds since 1Jan1904"=timestamp(3822521110.5518007 s since 1904-01-01), "mean[ps]"=42.94174194335943}, {"seconds since 1Jan1904"=timestamp(3822521411.9820223 s since 1904-01-01), "mean[ps]"=42.94174194335943}, {"seconds since 1Jan1904"=timestamp(3822521713.4490914 s since 1904-01-01), "mean[ps]"=42.94174194335943}, {"seconds since 1Jan1904"=timestamp(3822522014.93792 s since 1904-01-01), "mean[ps]"=42.4495788574219}, {"seconds since 1Jan1904"=timestamp(3822522316.3927464 s since 1904-01-01), "mean[ps]"=42.695660400390636}, {"seconds since 1Jan1904"=timestamp(3822522617.8067694 s since 1904-01-01), "mean[ps]"=42.695660400390636}, {"seconds since 1Jan1904"=timestamp(3822522919.2539024 s since 1904-01-01), "mean[ps]"=43.31086425781251}, {"seconds since 1Jan1904"=timestamp(3822523220.6865177 s since 1904-01-01), "mean[ps]"=43.06478271484377}, {"seconds since 1Jan1904"=timestamp(3822523522.1590304 s since 1904-01-01), "mean[ps]"=42.818701171875034}, {"seconds since 1Jan1904"=timestamp(3822523823.5384583 s since 1904-01-01), "mean[ps]"=42.20349731445316}, {"seconds since 1Jan1904"=timestamp(3822524124.9813824 s since 1904-01-01), "mean[ps]"=43.18782348632817}, {"seconds since 1Jan1904"=timestamp(3822524426.491788 s since 1904-01-01), "mean[ps]"=42.818701171875034}, {"seconds since 1Jan1904"=timestamp(3822524727.9125314 s since 1904-01-01), "mean[ps]"=42.94174194335943}, {"seconds since 1Jan1904"=timestamp(3822525029.379265 s since 1904-01-01), "mean[ps]"=42.818701171875034}, {"seconds since 1Jan1904"=timestamp(3822525330.781236 s since 1904-01-01), "mean[ps]"=43.55694580078131}, {"seconds since 1Jan1904"=timestamp(3822525632.329557 s since 1904-01-01), "mean[ps]"=43.31086425781251}, {"seconds since 1Jan1904"=timestamp(3822525933.784519 s since 1904-01-01), "mean[ps]"=42.94174194335943}, {"seconds since 1Jan1904"=timestamp(3822526235.2852225 s since 1904-01-01), "mean[ps]"=43.31086425781251}, {"seconds since 1Jan1904"=timestamp(3822526536.779774 s since 1904-01-01), "mean[ps]"=43.55694580078131}, {"seconds since 1Jan1904"=timestamp(3822526838.2156734 s since 1904-01-01), "mean[ps]"=43.43390502929691}, {"seconds since 1Jan1904"=timestamp(3822527139.721087 s since 1904-01-01), "mean[ps]"=43.18782348632817}, {"seconds since 1Jan1904"=timestamp(3822527441.1896977 s since 1904-01-01), "mean[ps]"=43.43390502929691}, {"seconds since 1Jan1904"=timestamp(3822527742.6183696 s since 1904-01-01), "mean[ps]"=43.18782348632817}, {"seconds since 1Jan1904"=timestamp(3822528044.0890102 s since 1904-01-01), "mean[ps]"=42.32653808593756}, {"seconds since 1Jan1904"=timestamp(3822528345.503568 s since 1904-01-01), "mean[ps]"=43.55694580078131}, {"seconds since 1Jan1904"=timestamp(3822528646.8947263 s since 1904-01-01), "mean[ps]"=43.18782348632817}, {"seconds since 1Jan1904"=timestamp(3822528948.387137 s since 1904-01-01), "mean[ps]"=43.55694580078131}, {"seconds since 1Jan1904"=timestamp(3822529249.822836 s since 1904-01-01), "mean[ps]"=43.43390502929691}, {"seconds since 1Jan1904"=timestamp(3822529551.2237015 s since 1904-01-01), "mean[ps]"=42.94174194335943}, {"seconds since 1Jan1904"=timestamp(3822529852.7132487 s since 1904-01-01), "mean[ps]"=43.31086425781251}, {"seconds since 1Jan1904"=timestamp(3822530154.13355 s since 1904-01-01), "mean[ps]"=43.55694580078131}, {"seconds since 1Jan1904"=timestamp(3822530455.5063615 s since 1904-01-01), "mean[ps]"=44.049108886718784}, {"seconds since 1Jan1904"=timestamp(3822530756.906737 s since 1904-01-01), "mean[ps]"=43.926068115234386}, {"seconds since 1Jan1904"=timestamp(3822531058.404439 s since 1904-01-01), "mean[ps]"=43.55694580078131}, {"seconds since 1Jan1904"=timestamp(3822531359.808485 s since 1904-01-01), "mean[ps]"=43.67998657226565}, {"seconds since 1Jan1904"=timestamp(3822531661.336039 s since 1904-01-01), "mean[ps]"=43.31086425781251}, {"seconds since 1Jan1904"=timestamp(3822531962.7850113 s since 1904-01-01), "mean[ps]"=43.06478271484377}, {"seconds since 1Jan1904"=timestamp(3822532264.2264094 s since 1904-01-01), "mean[ps]"=42.08045654296876}, {"seconds since 1Jan1904"=timestamp(3822532565.644325 s since 1904-01-01), "mean[ps]"=43.06478271484377}, {"seconds since 1Jan1904"=timestamp(3822532867.095218 s since 1904-01-01), "mean[ps]"=42.20349731445316}, {"seconds since 1Jan1904"=timestamp(3822533168.4954033 s since 1904-01-01), "mean[ps]"=42.08045654296876}, {"seconds since 1Jan1904"=timestamp(3822533470.0292826 s since 1904-01-01), "mean[ps]"=43.31086425781251}, {"seconds since 1Jan1904"=timestamp(3822533771.460639 s since 1904-01-01), "mean[ps]"=42.818701171875034}, {"seconds since 1Jan1904"=timestamp(3822534072.903432 s since 1904-01-01), "mean[ps]"=42.94174194335943}, {"seconds since 1Jan1904"=timestamp(3822534374.327941 s since 1904-01-01), "mean[ps]"=42.94174194335943}, {"seconds since 1Jan1904"=timestamp(3822534675.8510175 s since 1904-01-01), "mean[ps]"=42.572619628906295}, {"seconds since 1Jan1904"=timestamp(3822534977.3926754 s since 1904-01-01), "mean[ps]"=43.06478271484377}, {"seconds since 1Jan1904"=timestamp(3822535278.8113256 s since 1904-01-01), "mean[ps]"=43.31086425781251}, {"seconds since 1Jan1904"=timestamp(3822535580.052392 s since 1904-01-01), "mean[ps]"=42.695660400390636}, {"seconds since 1Jan1904"=timestamp(3822535881.6109457 s since 1904-01-01), "mean[ps]"=43.31086425781251}, {"seconds since 1Jan1904"=timestamp(3822536183.1016607 s since 1904-01-01), "mean[ps]"=42.08045654296876}, {"seconds since 1Jan1904"=timestamp(3822536484.4703193 s since 1904-01-01), "mean[ps]"=42.695660400390636}, {"seconds since 1Jan1904"=timestamp(3822536786.003652 s since 1904-01-01), "mean[ps]"=42.818701171875034}, {"seconds since 1Jan1904"=timestamp(3822537087.3877025 s since 1904-01-01), "mean[ps]"=42.32653808593756}, {"seconds since 1Jan1904"=timestamp(3822537388.9627695 s since 1904-01-01), "mean[ps]"=42.4495788574219}, {"seconds since 1Jan1904"=timestamp(3822537690.32478 s since 1904-01-01), "mean[ps]"=42.572619628906295}, {"seconds since 1Jan1904"=timestamp(3822537991.8736057 s since 1904-01-01), "mean[ps]"=42.32653808593756}, {"seconds since 1Jan1904"=timestamp(3822538293.281887 s since 1904-01-01), "mean[ps]"=42.818701171875034}, {"seconds since 1Jan1904"=timestamp(3822538594.700456 s since 1904-01-01), "mean[ps]"=42.695660400390636}, {"seconds since 1Jan1904"=timestamp(3822538896.2253175 s since 1904-01-01), "mean[ps]"=43.31086425781251}, {"seconds since 1Jan1904"=timestamp(3822539197.7020054 s since 1904-01-01), "mean[ps]"=42.572619628906295}, {"seconds since 1Jan1904"=timestamp(3822539499.1529503 s since 1904-01-01), "mean[ps]"=42.818701171875034}, {"seconds since 1Jan1904"=timestamp(3822539800.5176826 s since 1904-01-01), "mean[ps]"=42.818701171875034}, {"seconds since 1Jan1904"=timestamp(3822540101.955672 s since 1904-01-01), "mean[ps]"=42.818701171875034}, {"seconds since 1Jan1904"=timestamp(3822540403.389026 s since 1904-01-01), "mean[ps]"=42.08045654296876}, {"seconds since 1Jan1904"=timestamp(3822540704.8647823 s since 1904-01-01), "mean[ps]"=43.31086425781251}, {"seconds since 1Jan1904"=timestamp(3822541006.2905207 s since 1904-01-01), "mean[ps]"=43.43390502929691}, {"seconds since 1Jan1904"=timestamp(3822541307.8066297 s since 1904-01-01), "mean[ps]"=43.06478271484377}, {"seconds since 1Jan1904"=timestamp(3822541609.3079934 s since 1904-01-01), "mean[ps]"=42.94174194335943}, {"seconds since 1Jan1904"=timestamp(3822541910.788964 s since 1904-01-01), "mean[ps]"=42.20349731445316}, {"seconds since 1Jan1904"=timestamp(3822542212.360313 s since 1904-01-01), "mean[ps]"=42.572619628906295}, {"seconds since 1Jan1904"=timestamp(3822542513.8452806 s since 1904-01-01), "mean[ps]"=43.31086425781251}, {"seconds since 1Jan1904"=timestamp(3822542815.328869 s since 1904-01-01), "mean[ps]"=42.4495788574219}, {"seconds since 1Jan1904"=timestamp(3822543116.8031616 s since 1904-01-01), "mean[ps]"=42.08045654296876}, {"seconds since 1Jan1904"=timestamp(3822543418.253579 s since 1904-01-01), "mean[ps]"=10.828100585937534}, {"seconds since 1Jan1904"=timestamp(3822543719.8005633 s since 1904-01-01), "mean[ps]"=43.06478271484377}, {"seconds since 1Jan1904"=timestamp(3822544021.284577 s since 1904-01-01), "mean[ps]"=42.94174194335943}, {"seconds since 1Jan1904"=timestamp(3822544322.8030105 s since 1904-01-01), "mean[ps]"=42.94174194335943}, {"seconds since 1Jan1904"=timestamp(3822544624.2975945 s since 1904-01-01), "mean[ps]"=42.695660400390636}, {"seconds since 1Jan1904"=timestamp(3822544925.818383 s since 1904-01-01), "mean[ps]"=43.06478271484377}, {"seconds since 1Jan1904"=timestamp(3822545227.2305446 s since 1904-01-01), "mean[ps]"=42.818701171875034}, {"seconds since 1Jan1904"=timestamp(3822545528.6374345 s since 1904-01-01), "mean[ps]"=42.695660400390636}, {"seconds since 1Jan1904"=timestamp(3822545830.161919 s since 1904-01-01), "mean[ps]"=42.20349731445316}, {"seconds since 1Jan1904"=timestamp(3822546131.6581616 s since 1904-01-01), "mean[ps]"=43.06478271484377}, {"seconds since 1Jan1904"=timestamp(3822546433.1208367 s since 1904-01-01), "mean[ps]"=42.94174194335943}, {"seconds since 1Jan1904"=timestamp(3822546734.5235424 s since 1904-01-01), "mean[ps]"=42.695660400390636}, {"seconds since 1Jan1904"=timestamp(3822547035.9215217 s since 1904-01-01), "mean[ps]"=42.94174194335943}, {"seconds since 1Jan1904"=timestamp(3822547337.4649706 s since 1904-01-01), "mean[ps]"=43.43390502929691}, {"seconds since 1Jan1904"=timestamp(3822547638.88064 s since 1904-01-01), "mean[ps]"=42.695660400390636}, {"seconds since 1Jan1904"=timestamp(3822547940.3121905 s since 1904-01-01), "mean[ps]"=42.695660400390636}, {"seconds since 1Jan1904"=timestamp(3822548241.74978 s since 1904-01-01), "mean[ps]"=41.95741577148442}, {"seconds since 1Jan1904"=timestamp(3822548543.2799606 s since 1904-01-01), "mean[ps]"=42.818701171875034}, {"seconds since 1Jan1904"=timestamp(3822548844.742632 s since 1904-01-01), "mean[ps]"=42.695660400390636}, {"seconds since 1Jan1904"=timestamp(3822549146.149104 s since 1904-01-01), "mean[ps]"=42.4495788574219}, {"seconds since 1Jan1904"=timestamp(3822549447.533661 s since 1904-01-01), "mean[ps]"=42.4495788574219}, {"seconds since 1Jan1904"=timestamp(3822549748.9579425 s since 1904-01-01), "mean[ps]"=42.695660400390636}, {"seconds since 1Jan1904"=timestamp(3822550050.4716654 s since 1904-01-01), "mean[ps]"=41.95741577148442}, {"seconds since 1Jan1904"=timestamp(3822550351.947339 s since 1904-01-01), "mean[ps]"=42.572619628906295}, {"seconds since 1Jan1904"=timestamp(3822550653.458123 s since 1904-01-01), "mean[ps]"=41.95741577148442}, {"seconds since 1Jan1904"=timestamp(3822550954.99518 s since 1904-01-01), "mean[ps]"=42.572619628906295}, {"seconds since 1Jan1904"=timestamp(3822551256.5036974 s since 1904-01-01), "mean[ps]"=42.818701171875034}, {"seconds since 1Jan1904"=timestamp(3822551558.0137887 s since 1904-01-01), "mean[ps]"=42.4495788574219}, {"seconds since 1Jan1904"=timestamp(3822551859.5051265 s since 1904-01-01), "mean[ps]"=42.695660400390636}, {"seconds since 1Jan1904"=timestamp(3822552161.039615 s since 1904-01-01), "mean[ps]"=42.94174194335943}, {"seconds since 1Jan1904"=timestamp(3822552462.609901 s since 1904-01-01), "mean[ps]"=42.4495788574219}, {"seconds since 1Jan1904"=timestamp(3822552764.000548 s since 1904-01-01), "mean[ps]"=42.4495788574219}, {"seconds since 1Jan1904"=timestamp(3822553065.419496 s since 1904-01-01), "mean[ps]"=42.572619628906295}, {"seconds since 1Jan1904"=timestamp(3822553366.9214015 s since 1904-01-01), "mean[ps]"=43.31086425781251}, {"seconds since 1Jan1904"=timestamp(3822553668.2656054 s since 1904-01-01), "mean[ps]"=42.32653808593756}, {"seconds since 1Jan1904"=timestamp(3822553969.7844114 s since 1904-01-01), "mean[ps]"=42.695660400390636}, {"seconds since 1Jan1904"=timestamp(3822554271.2343993 s since 1904-01-01), "mean[ps]"=42.818701171875034}, {"seconds since 1Jan1904"=timestamp(3822554572.7825623 s since 1904-01-01), "mean[ps]"=42.94174194335943}, {"seconds since 1Jan1904"=timestamp(3822554874.2372446 s since 1904-01-01), "mean[ps]"=43.31086425781251}, {"seconds since 1Jan1904"=timestamp(3822555175.792369 s since 1904-01-01), "mean[ps]"=42.572619628906295}, {"seconds since 1Jan1904"=timestamp(3822555477.2372074 s since 1904-01-01), "mean[ps]"=42.94174194335943}, {"seconds since 1Jan1904"=timestamp(3822555778.701035 s since 1904-01-01), "mean[ps]"=43.43390502929691}, {"seconds since 1Jan1904"=timestamp(3822556080.2516418 s since 1904-01-01), "mean[ps]"=42.4495788574219}, {"seconds since 1Jan1904"=timestamp(3822556381.757804 s since 1904-01-01), "mean[ps]"=42.572619628906295}, {"seconds since 1Jan1904"=timestamp(3822556683.148675 s since 1904-01-01), "mean[ps]"=42.572619628906295}, {"seconds since 1Jan1904"=timestamp(3822556984.6444607 s since 1904-01-01), "mean[ps]"=43.803027343750045}, {"seconds since 1Jan1904"=timestamp(3822557286.095585 s since 1904-01-01), "mean[ps]"=42.32653808593756}, {"seconds since 1Jan1904"=timestamp(3822557587.5588975 s since 1904-01-01), "mean[ps]"=42.695660400390636}, {"seconds since 1Jan1904"=timestamp(3822557889.0395904 s since 1904-01-01), "mean[ps]"=43.06478271484377}, {"seconds since 1Jan1904"=timestamp(3822558190.4474607 s since 1904-01-01), "mean[ps]"=42.94174194335943}, {"seconds since 1Jan1904"=timestamp(3822558492.0190606 s since 1904-01-01), "mean[ps]"=42.94174194335943}, {"seconds since 1Jan1904"=timestamp(3822558793.477814 s since 1904-01-01), "mean[ps]"=42.818701171875034}, {"seconds since 1Jan1904"=timestamp(3822559094.921321 s since 1904-01-01), "mean[ps]"=42.94174194335943}, {"seconds since 1Jan1904"=timestamp(3822559396.4460673 s since 1904-01-01), "mean[ps]"=42.818701171875034}, {"seconds since 1Jan1904"=timestamp(3822559697.9183455 s since 1904-01-01), "mean[ps]"=43.18782348632817}, {"seconds since 1Jan1904"=timestamp(3822559999.3983808 s since 1904-01-01), "mean[ps]"=41.83437500000002}, {"seconds since 1Jan1904"=timestamp(3822560300.8987856 s since 1904-01-01), "mean[ps]"=42.20349731445316}, {"seconds since 1Jan1904"=timestamp(3822560602.3556256 s since 1904-01-01), "mean[ps]"=42.572619628906295}, {"seconds since 1Jan1904"=timestamp(3822560903.899011 s since 1904-01-01), "mean[ps]"=43.06478271484377}, {"seconds since 1Jan1904"=timestamp(3822561205.442392 s since 1904-01-01), "mean[ps]"=42.08045654296876}, {"seconds since 1Jan1904"=timestamp(3822561506.864459 s since 1904-01-01), "mean[ps]"=42.818701171875034}, {"seconds since 1Jan1904"=timestamp(3822561808.4265895 s since 1904-01-01), "mean[ps]"=43.55694580078131}, {"seconds since 1Jan1904"=timestamp(3822562109.9678545 s since 1904-01-01), "mean[ps]"=42.818701171875034}, {"seconds since 1Jan1904"=timestamp(3822562411.5341334 s since 1904-01-01), "mean[ps]"=42.4495788574219}, {"seconds since 1Jan1904"=timestamp(3822562712.998142 s since 1904-01-01), "mean[ps]"=43.43390502929691}, {"seconds since 1Jan1904"=timestamp(3822563014.480204 s since 1904-01-01), "mean[ps]"=43.18782348632817}, {"seconds since 1Jan1904"=timestamp(3822563315.9980226 s since 1904-01-01), "mean[ps]"=41.95741577148442}, {"seconds since 1Jan1904"=timestamp(3822563617.240683 s since 1904-01-01), "mean[ps]"=41.95741577148442}, {"seconds since 1Jan1904"=timestamp(3822563918.749057 s since 1904-01-01), "mean[ps]"=42.818701171875034}, {"seconds since 1Jan1904"=timestamp(3822564220.254855 s since 1904-01-01), "mean[ps]"=42.695660400390636}, {"seconds since 1Jan1904"=timestamp(3822564521.8313217 s since 1904-01-01), "mean[ps]"=42.818701171875034}, {"seconds since 1Jan1904"=timestamp(3822564823.2753153 s since 1904-01-01), "mean[ps]"=42.572619628906295}, {"seconds since 1Jan1904"=timestamp(3822565124.701639 s since 1904-01-01), "mean[ps]"=43.31086425781251}, {"seconds since 1Jan1904"=timestamp(3822565426.1726537 s since 1904-01-01), "mean[ps]"=42.818701171875034}, {"seconds since 1Jan1904"=timestamp(3822565727.6830926 s since 1904-01-01), "mean[ps]"=42.4495788574219}, {"seconds since 1Jan1904"=timestamp(3822566029.165819 s since 1904-01-01), "mean[ps]"=42.695660400390636}, {"seconds since 1Jan1904"=timestamp(3822566330.740963 s since 1904-01-01), "mean[ps]"=42.4495788574219}, {"seconds since 1Jan1904"=timestamp(3822566632.249509 s since 1904-01-01), "mean[ps]"=43.18782348632817}, {"seconds since 1Jan1904"=timestamp(3822566933.704676 s since 1904-01-01), "mean[ps]"=42.572619628906295}, {"seconds since 1Jan1904"=timestamp(3822567235.209213 s since 1904-01-01), "mean[ps]"=42.4495788574219}, {"seconds since 1Jan1904"=timestamp(3822567536.6946225 s since 1904-01-01), "mean[ps]"=42.32653808593756}, {"seconds since 1Jan1904"=timestamp(3822567838.169631 s since 1904-01-01), "mean[ps]"=42.94174194335943}, {"seconds since 1Jan1904"=timestamp(3822568139.6286063 s since 1904-01-01), "mean[ps]"=41.83437500000002}, {"seconds since 1Jan1904"=timestamp(3822568441.096488 s since 1904-01-01), "mean[ps]"=42.32653808593756}, {"seconds since 1Jan1904"=timestamp(3822568742.5332594 s since 1904-01-01), "mean[ps]"=43.06478271484377}, {"seconds since 1Jan1904"=timestamp(3822569044.0896015 s since 1904-01-01), "mean[ps]"=42.94174194335943}, {"seconds since 1Jan1904"=timestamp(3822569345.551961 s since 1904-01-01), "mean[ps]"=42.4495788574219}, {"seconds since 1Jan1904"=timestamp(3822569647.024821 s since 1904-01-01), "mean[ps]"=42.4495788574219}, {"seconds since 1Jan1904"=timestamp(3822569948.559713 s since 1904-01-01), "mean[ps]"=73.20977172851565}, {"seconds since 1Jan1904"=timestamp(3822570249.9499383 s since 1904-01-01), "mean[ps]"=42.4495788574219}, {"seconds since 1Jan1904"=timestamp(3822570551.4543366 s since 1904-01-01), "mean[ps]"=42.32653808593756}, {"seconds since 1Jan1904"=timestamp(3822570852.907388 s since 1904-01-01), "mean[ps]"=42.94174194335943}, {"seconds since 1Jan1904"=timestamp(3822571154.3613434 s since 1904-01-01), "mean[ps]"=42.20349731445316}, {"seconds since 1Jan1904"=timestamp(3822571455.875889 s since 1904-01-01), "mean[ps]"=42.32653808593756}, {"seconds since 1Jan1904"=timestamp(3822571757.4035335 s since 1904-01-01), "mean[ps]"=42.08045654296876}, {"seconds since 1Jan1904"=timestamp(3822572058.8738127 s since 1904-01-01), "mean[ps]"=10.951141357421932}, {"seconds since 1Jan1904"=timestamp(3822572360.3478255 s since 1904-01-01), "mean[ps]"=42.695660400390636}, {"seconds since 1Jan1904"=timestamp(3822572661.834789 s since 1904-01-01), "mean[ps]"=42.572619628906295}, {"seconds since 1Jan1904"=timestamp(3822572963.3136296 s since 1904-01-01), "mean[ps]"=42.695660400390636}, {"seconds since 1Jan1904"=timestamp(3822573264.8089194 s since 1904-01-01), "mean[ps]"=42.08045654296876}, {"seconds since 1Jan1904"=timestamp(3822573566.2905793 s since 1904-01-01), "mean[ps]"=42.08045654296876}, {"seconds since 1Jan1904"=timestamp(3822573867.753861 s since 1904-01-01), "mean[ps]"=42.4495788574219}, {"seconds since 1Jan1904"=timestamp(3822574169.3307586 s since 1904-01-01), "mean[ps]"=73.20977172851565}, {"seconds since 1Jan1904"=timestamp(3822574470.7852354 s since 1904-01-01), "mean[ps]"=43.06478271484377}, {"seconds since 1Jan1904"=timestamp(3822574772.1922865 s since 1904-01-01), "mean[ps]"=42.08045654296876}, {"seconds since 1Jan1904"=timestamp(3822575073.6485744 s since 1904-01-01), "mean[ps]"=41.83437500000002}, {"seconds since 1Jan1904"=timestamp(3822575375.0628457 s since 1904-01-01), "mean[ps]"=42.572619628906295}, {"seconds since 1Jan1904"=timestamp(3822575676.540885 s since 1904-01-01), "mean[ps]"=42.20349731445316}, {"seconds since 1Jan1904"=timestamp(3822575978.110875 s since 1904-01-01), "mean[ps]"=42.695660400390636}, {"seconds since 1Jan1904"=timestamp(3822576279.6679864 s since 1904-01-01), "mean[ps]"=42.32653808593756}, {"seconds since 1Jan1904"=timestamp(3822576581.2032743 s since 1904-01-01), "mean[ps]"=42.32653808593756}, {"seconds since 1Jan1904"=timestamp(3822576882.6405673 s since 1904-01-01), "mean[ps]"=41.83437500000002}, {"seconds since 1Jan1904"=timestamp(3822577184.1204553 s since 1904-01-01), "mean[ps]"=42.32653808593756}, {"seconds since 1Jan1904"=timestamp(3822577485.6404696 s since 1904-01-01), "mean[ps]"=43.06478271484377}, {"seconds since 1Jan1904"=timestamp(3822577787.095057 s since 1904-01-01), "mean[ps]"=42.818701171875034}, {"seconds since 1Jan1904"=timestamp(3822578088.553026 s since 1904-01-01), "mean[ps]"=42.818701171875034}, {"seconds since 1Jan1904"=timestamp(3822578390.115008 s since 1904-01-01), "mean[ps]"=42.4495788574219}, {"seconds since 1Jan1904"=timestamp(3822578691.551293 s since 1904-01-01), "mean[ps]"=42.08045654296876}, {"seconds since 1Jan1904"=timestamp(3822578992.9199705 s since 1904-01-01), "mean[ps]"=42.20349731445316}, {"seconds since 1Jan1904"=timestamp(3822579294.3933854 s since 1904-01-01), "mean[ps]"=41.95741577148442}, {"seconds since 1Jan1904"=timestamp(3822579595.918991 s since 1904-01-01), "mean[ps]"=42.20349731445316}, {"seconds since 1Jan1904"=timestamp(3822579897.4222097 s since 1904-01-01), "mean[ps]"=42.08045654296876}, {"seconds since 1Jan1904"=timestamp(3822580198.9128265 s since 1904-01-01), "mean[ps]"=73.20977172851565}, {"seconds since 1Jan1904"=timestamp(3822580500.314174 s since 1904-01-01), "mean[ps]"=41.83437500000002}, {"seconds since 1Jan1904"=timestamp(3822580801.8501215 s since 1904-01-01), "mean[ps]"=42.695660400390636}, {"seconds since 1Jan1904"=timestamp(3822581103.3778 s since 1904-01-01), "mean[ps]"=42.695660400390636}, {"seconds since 1Jan1904"=timestamp(3822581404.880745 s since 1904-01-01), "mean[ps]"=73.20977172851565}, {"seconds since 1Jan1904"=timestamp(3822581706.4360175 s since 1904-01-01), "mean[ps]"=42.20349731445316}, {"seconds since 1Jan1904"=timestamp(3822582007.8203206 s since 1904-01-01), "mean[ps]"=42.32653808593756}, {"seconds since 1Jan1904"=timestamp(3822582309.2484713 s since 1904-01-01), "mean[ps]"=42.20349731445316}, {"seconds since 1Jan1904"=timestamp(3822582610.7182074 s since 1904-01-01), "mean[ps]"=41.95741577148442}, {"seconds since 1Jan1904"=timestamp(3822582912.221481 s since 1904-01-01), "mean[ps]"=41.588293457031284}, {"seconds since 1Jan1904"=timestamp(3822583213.701206 s since 1904-01-01), "mean[ps]"=42.20349731445316}, {"seconds since 1Jan1904"=timestamp(3822583515.2400217 s since 1904-01-01), "mean[ps]"=10.582019042968795}, {"seconds since 1Jan1904"=timestamp(3822583816.7411456 s since 1904-01-01), "mean[ps]"=42.08045654296876}, {"seconds since 1Jan1904"=timestamp(3822584118.2147617 s since 1904-01-01), "mean[ps]"=41.83437500000002}, {"seconds since 1Jan1904"=timestamp(3822584419.675927 s since 1904-01-01), "mean[ps]"=10.582019042968795}, {"seconds since 1Jan1904"=timestamp(3822584721.0923023 s since 1904-01-01), "mean[ps]"=73.0867309570313}, {"seconds since 1Jan1904"=timestamp(3822585022.5496383 s since 1904-01-01), "mean[ps]"=41.342211914062545}, {"seconds since 1Jan1904"=timestamp(3822585324.043527 s since 1904-01-01), "mean[ps]"=41.83437500000002}, {"seconds since 1Jan1904"=timestamp(3822585625.471996 s since 1904-01-01), "mean[ps]"=42.4495788574219}, {"seconds since 1Jan1904"=timestamp(3822585926.8942423 s since 1904-01-01), "mean[ps]"=73.20977172851565}, {"seconds since 1Jan1904"=timestamp(3822586228.3225694 s since 1904-01-01), "mean[ps]"=41.588293457031284}, {"seconds since 1Jan1904"=timestamp(3822586529.8338766 s since 1904-01-01), "mean[ps]"=10.582019042968795}, {"seconds since 1Jan1904"=timestamp(3822586831.2920294 s since 1904-01-01), "mean[ps]"=41.95741577148442}, {"seconds since 1Jan1904"=timestamp(3822587132.7088814 s since 1904-01-01), "mean[ps]"=41.95741577148442}, {"seconds since 1Jan1904"=timestamp(3822587434.1071906 s since 1904-01-01), "mean[ps]"=42.32653808593756}, {"seconds since 1Jan1904"=timestamp(3822587735.3207207 s since 1904-01-01), "mean[ps]"=73.0867309570313}, {"seconds since 1Jan1904"=timestamp(3822588036.7855854 s since 1904-01-01), "mean[ps]"=42.08045654296876}, {"seconds since 1Jan1904"=timestamp(3822588338.3446593 s since 1904-01-01), "mean[ps]"=72.84064941406251}, {"seconds since 1Jan1904"=timestamp(3822588639.839839 s since 1904-01-01), "mean[ps]"=41.83437500000002}, {"seconds since 1Jan1904"=timestamp(3822588941.288984 s since 1904-01-01), "mean[ps]"=42.20349731445316}, {"seconds since 1Jan1904"=timestamp(3822589242.7402463 s since 1904-01-01), "mean[ps]"=73.0867309570313}, {"seconds since 1Jan1904"=timestamp(3822589544.2098656 s since 1904-01-01), "mean[ps]"=42.08045654296876}, {"seconds since 1Jan1904"=timestamp(3822589845.6971216 s since 1904-01-01), "mean[ps]"=42.32653808593756}, {"seconds since 1Jan1904"=timestamp(3822590147.2125216 s since 1904-01-01), "mean[ps]"=10.828100585937534}, {"seconds since 1Jan1904"=timestamp(3822590448.640258 s since 1904-01-01), "mean[ps]"=10.582019042968795}, {"seconds since 1Jan1904"=timestamp(3822590750.1391034 s since 1904-01-01), "mean[ps]"=10.335937500000057}, {"seconds since 1Jan1904"=timestamp(3822591051.5836415 s since 1904-01-01), "mean[ps]"=41.71133422851568}, {"seconds since 1Jan1904"=timestamp(3822591352.9831247 s since 1904-01-01), "mean[ps]"=42.572619628906295}, {"seconds since 1Jan1904"=timestamp(3822591654.485979 s since 1904-01-01), "mean[ps]"=10.335937500000057}, {"seconds since 1Jan1904"=timestamp(3822591955.859042 s since 1904-01-01), "mean[ps]"=41.95741577148442}, {"seconds since 1Jan1904"=timestamp(3822592257.408669 s since 1904-01-01), "mean[ps]"=73.20977172851565}, {"seconds since 1Jan1904"=timestamp(3822592558.932187 s since 1904-01-01), "mean[ps]"=41.342211914062545}, {"seconds since 1Jan1904"=timestamp(3822592860.391513 s since 1904-01-01), "mean[ps]"=41.83437500000002}, {"seconds since 1Jan1904"=timestamp(3822593161.860652 s since 1904-01-01), "mean[ps]"=41.21917114257815}, {"seconds since 1Jan1904"=timestamp(3822593463.385323 s since 1904-01-01), "mean[ps]"=42.572619628906295}, {"seconds since 1Jan1904"=timestamp(3822593764.8500686 s since 1904-01-01), "mean[ps]"=72.96369018554691}, {"seconds since 1Jan1904"=timestamp(3822594066.308588 s since 1904-01-01), "mean[ps]"=41.21917114257815}, {"seconds since 1Jan1904"=timestamp(3822594367.780607 s since 1904-01-01), "mean[ps]"=10.458978271484398}, {"seconds since 1Jan1904"=timestamp(3822594669.2577024 s since 1904-01-01), "mean[ps]"=42.08045654296876}, {"seconds since 1Jan1904"=timestamp(3822594970.726291 s since 1904-01-01), "mean[ps]"=10.582019042968795}, {"seconds since 1Jan1904"=timestamp(3822595272.1390114 s since 1904-01-01), "mean[ps]"=10.582019042968795}, {"seconds since 1Jan1904"=timestamp(3822595573.6779704 s since 1904-01-01), "mean[ps]"=41.342211914062545}, {"seconds since 1Jan1904"=timestamp(3822595875.2007656 s since 1904-01-01), "mean[ps]"=41.342211914062545}, {"seconds since 1Jan1904"=timestamp(3822596176.6578298 s since 1904-01-01), "mean[ps]"=73.20977172851565}, {"seconds since 1Jan1904"=timestamp(3822596478.2190976 s since 1904-01-01), "mean[ps]"=73.0867309570313}, {"seconds since 1Jan1904"=timestamp(3822596779.7422447 s since 1904-01-01), "mean[ps]"=41.83437500000002}, {"seconds since 1Jan1904"=timestamp(3822597081.1809144 s since 1904-01-01), "mean[ps]"=41.83437500000002}, {"seconds since 1Jan1904"=timestamp(3822597382.686327 s since 1904-01-01), "mean[ps]"=72.84064941406251}, {"seconds since 1Jan1904"=timestamp(3822597684.2478952 s since 1904-01-01), "mean[ps]"=41.71133422851568}, {"seconds since 1Jan1904"=timestamp(3822597985.7226458 s since 1904-01-01), "mean[ps]"=42.20349731445316}, {"seconds since 1Jan1904"=timestamp(3822598287.212348 s since 1904-01-01), "mean[ps]"=10.458978271484398}, {"seconds since 1Jan1904"=timestamp(3822598588.6026154 s since 1904-01-01), "mean[ps]"=41.71133422851568}, {"seconds since 1Jan1904"=timestamp(3822598890.0572553 s since 1904-01-01), "mean[ps]"=42.32653808593756}, {"seconds since 1Jan1904"=timestamp(3822599191.425584 s since 1904-01-01), "mean[ps]"=42.32653808593756}, {"seconds since 1Jan1904"=timestamp(3822599492.866769 s since 1904-01-01), "mean[ps]"=42.818701171875034}, {"seconds since 1Jan1904"=timestamp(3822599794.2904983 s since 1904-01-01), "mean[ps]"=42.695660400390636}, {"seconds since 1Jan1904"=timestamp(3822600095.7871695 s since 1904-01-01), "mean[ps]"=43.18782348632817}, {"seconds since 1Jan1904"=timestamp(3822600397.4508214 s since 1904-01-01), "mean[ps]"=43.67998657226565}, {"seconds since 1Jan1904"=timestamp(3822600698.83722 s since 1904-01-01), "mean[ps]"=43.67998657226565}, {"seconds since 1Jan1904"=timestamp(3822601000.21038 s since 1904-01-01), "mean[ps]"=43.31086425781251}, {"seconds since 1Jan1904"=timestamp(3822601301.7260976 s since 1904-01-01), "mean[ps]"=42.94174194335943}]
  in  "stop":bool
  out "误差线":refnum<class "2D Plot Datatype.lvclass">[](xcontrol)
  out "sigma[ps]":dbl=47.77065519923074 format="%0.2f"
  out "Sigma":T1(graph)=[{"seconds since 1Jan1904"=timestamp(3822506942.315674 s since 1904-01-01), "mean[ps]"=48.159483831069075}, {"seconds since 1Jan1904"=timestamp(3822507243.6711025 s since 1904-01-01), "mean[ps]"=47.408858847112896}, {"seconds since 1Jan1904"=timestamp(3822507545.1626496 s since 1904-01-01), "mean[ps]"=46.61942019456449}, {"seconds since 1Jan1904"=timestamp(3822507846.553396 s since 1904-01-01), "mean[ps]"=48.80667678227107}, {"seconds since 1Jan1904"=timestamp(3822508148.061275 s since 1904-01-01), "mean[ps]"=49.06268181740717}, {"seconds since 1Jan1904"=timestamp(3822508449.501727 s since 1904-01-01), "mean[ps]"=46.182665671236094}, {"seconds since 1Jan1904"=timestamp(3822508750.8988624 s since 1904-01-01), "mean[ps]"=46.257724210817486}, {"seconds since 1Jan1904"=timestamp(3822509052.3161006 s since 1904-01-01), "mean[ps]"=47.361287211332396}, {"seconds since 1Jan1904"=timestamp(3822509353.734636 s since 1904-01-01), "mean[ps]"=46.9480186455856}, {"seconds since 1Jan1904"=timestamp(3822509655.1987686 s since 1904-01-01), "mean[ps]"=45.8920152517327}, {"seconds since 1Jan1904"=timestamp(3822509956.4995074 s since 1904-01-01), "mean[ps]"=45.57451643915388}, {"seconds since 1Jan1904"=timestamp(3822510257.982245 s since 1904-01-01), "mean[ps]"=47.315463385167625}, {"seconds since 1Jan1904"=timestamp(3822510559.3960705 s since 1904-01-01), "mean[ps]"=47.90140759346258}, {"seconds since 1Jan1904"=timestamp(3822510860.7242055 s since 1904-01-01), "mean[ps]"=47.479309403675536}, {"seconds since 1Jan1904"=timestamp(3822511162.215253 s since 1904-01-01), "mean[ps]"=47.782254006683296}, {"seconds since 1Jan1904"=timestamp(3822511463.639548 s since 1904-01-01), "mean[ps]"=46.161337675343326}, {"seconds since 1Jan1904"=timestamp(3822511765.766084 s since 1904-01-01), "mean[ps]"=50.49369984050864}, {"seconds since 1Jan1904"=timestamp(3822512067.2562017 s since 1904-01-01), "mean[ps]"=47.834485277452984}, {"seconds since 1Jan1904"=timestamp(3822512368.655607 s since 1904-01-01), "mean[ps]"=49.02557216238062}, {"seconds since 1Jan1904"=timestamp(3822512670.1464553 s since 1904-01-01), "mean[ps]"=45.814166398368876}, {"seconds since 1Jan1904"=timestamp(3822512971.507803 s since 1904-01-01), "mean[ps]"=48.51653742403675}, {"seconds since 1Jan1904"=timestamp(3822513272.925895 s since 1904-01-01), "mean[ps]"=46.680756118951976}, {"seconds since 1Jan1904"=timestamp(3822513574.303528 s since 1904-01-01), "mean[ps]"=48.41262836960416}, {"seconds since 1Jan1904"=timestamp(3822513875.706833 s since 1904-01-01), "mean[ps]"=47.97550750733224}, {"seconds since 1Jan1904"=timestamp(3822514177.255216 s since 1904-01-01), "mean[ps]"=45.89545932368381}, {"seconds since 1Jan1904"=timestamp(3822514478.6136312 s since 1904-01-01), "mean[ps]"=49.90310620710574}, {"seconds since 1Jan1904"=timestamp(3822514780.1012654 s since 1904-01-01), "mean[ps]"=47.55092179900368}, {"seconds since 1Jan1904"=timestamp(3822515081.6113095 s since 1904-01-01), "mean[ps]"=48.39744885609497}, {"seconds since 1Jan1904"=timestamp(3822515382.9461207 s since 1904-01-01), "mean[ps]"=48.28734698250283}, {"seconds since 1Jan1904"=timestamp(3822515684.3828025 s since 1904-01-01), "mean[ps]"=47.87117529033718}, {"seconds since 1Jan1904"=timestamp(3822515985.8758097 s since 1904-01-01), "mean[ps]"=49.262283167789505}, {"seconds since 1Jan1904"=timestamp(3822516287.3353777 s since 1904-01-01), "mean[ps]"=47.22916799702066}, {"seconds since 1Jan1904"=timestamp(3822516588.8038144 s since 1904-01-01), "mean[ps]"=48.50037095899462}, {"seconds since 1Jan1904"=timestamp(3822516890.2282143 s since 1904-01-01), "mean[ps]"=48.53953929089988}, {"seconds since 1Jan1904"=timestamp(3822517191.6262407 s since 1904-01-01), "mean[ps]"=48.2181292090042}, {"seconds since 1Jan1904"=timestamp(3822517493.0924606 s since 1904-01-01), "mean[ps]"=46.01944040425869}, {"seconds since 1Jan1904"=timestamp(3822517794.532418 s since 1904-01-01), "mean[ps]"=48.611784773270934}, {"seconds since 1Jan1904"=timestamp(3822518095.958946 s since 1904-01-01), "mean[ps]"=47.85829210085147}, {"seconds since 1Jan1904"=timestamp(3822518397.3720393 s since 1904-01-01), "mean[ps]"=47.19204546946518}, {"seconds since 1Jan1904"=timestamp(3822518698.777503 s since 1904-01-01), "mean[ps]"=47.71714397503429}, {"seconds since 1Jan1904"=timestamp(3822519000.1937714 s since 1904-01-01), "mean[ps]"=47.83596188508312}, {"seconds since 1Jan1904"=timestamp(3822519301.6194086 s since 1904-01-01), "mean[ps]"=46.64811173902966}, {"seconds since 1Jan1904"=timestamp(3822519603.042124 s since 1904-01-01), "mean[ps]"=47.91861049406198}, {"seconds since 1Jan1904"=timestamp(3822519904.578883 s since 1904-01-01), "mean[ps]"=49.14380526557847}, {"seconds since 1Jan1904"=timestamp(3822520206.0544343 s since 1904-01-01), "mean[ps]"=47.91867269370284}, {"seconds since 1Jan1904"=timestamp(3822520507.509728 s since 1904-01-01), "mean[ps]"=49.01199759799499}, {"seconds since 1Jan1904"=timestamp(3822520809.0371656 s since 1904-01-01), "mean[ps]"=47.67775817585235}, {"seconds since 1Jan1904"=timestamp(3822521110.5518007 s since 1904-01-01), "mean[ps]"=49.398401788916}, {"seconds since 1Jan1904"=timestamp(3822521411.9820223 s since 1904-01-01), "mean[ps]"=48.51677048788343}, {"seconds since 1Jan1904"=timestamp(3822521713.4490914 s since 1904-01-01), "mean[ps]"=48.49286633570731}, {"seconds since 1Jan1904"=timestamp(3822522014.93792 s since 1904-01-01), "mean[ps]"=47.05829962329567}, {"seconds since 1Jan1904"=timestamp(3822522316.3927464 s since 1904-01-01), "mean[ps]"=47.32587689000402}, {"seconds since 1Jan1904"=timestamp(3822522617.8067694 s since 1904-01-01), "mean[ps]"=48.38569192385885}, {"seconds since 1Jan1904"=timestamp(3822522919.2539024 s since 1904-01-01), "mean[ps]"=47.32009120074914}, {"seconds since 1Jan1904"=timestamp(3822523220.6865177 s since 1904-01-01), "mean[ps]"=46.27685463105682}, {"seconds since 1Jan1904"=timestamp(3822523522.1590304 s since 1904-01-01), "mean[ps]"=45.709177137160424}, {"seconds since 1Jan1904"=timestamp(3822523823.5384583 s since 1904-01-01), "mean[ps]"=48.782787729707586}, {"seconds since 1Jan1904"=timestamp(3822524124.9813824 s since 1904-01-01), "mean[ps]"=47.293404686818704}, {"seconds since 1Jan1904"=timestamp(3822524426.491788 s since 1904-01-01), "mean[ps]"=48.25510232004328}, {"seconds since 1Jan1904"=timestamp(3822524727.9125314 s since 1904-01-01), "mean[ps]"=46.90155284058185}, {"seconds since 1Jan1904"=timestamp(3822525029.379265 s since 1904-01-01), "mean[ps]"=46.486884169737344}, {"seconds since 1Jan1904"=timestamp(3822525330.781236 s since 1904-01-01), "mean[ps]"=45.57848080436541}, {"seconds since 1Jan1904"=timestamp(3822525632.329557 s since 1904-01-01), "mean[ps]"=47.06606685122013}, {"seconds since 1Jan1904"=timestamp(3822525933.784519 s since 1904-01-01), "mean[ps]"=45.33655821170527}, {"seconds since 1Jan1904"=timestamp(3822526235.2852225 s since 1904-01-01), "mean[ps]"=47.63570357584454}, {"seconds since 1Jan1904"=timestamp(3822526536.779774 s since 1904-01-01), "mean[ps]"=48.01285593423697}, {"seconds since 1Jan1904"=timestamp(3822526838.2156734 s since 1904-01-01), "mean[ps]"=47.09535161997451}, {"seconds since 1Jan1904"=timestamp(3822527139.721087 s since 1904-01-01), "mean[ps]"=47.374605843179324}, {"seconds since 1Jan1904"=timestamp(3822527441.1896977 s since 1904-01-01), "mean[ps]"=48.09953512727775}, {"seconds since 1Jan1904"=timestamp(3822527742.6183696 s since 1904-01-01), "mean[ps]"=48.46416984883609}, {"seconds since 1Jan1904"=timestamp(3822528044.0890102 s since 1904-01-01), "mean[ps]"=45.679923482515925}, {"seconds since 1Jan1904"=timestamp(3822528345.503568 s since 1904-01-01), "mean[ps]"=47.52658300576498}, {"seconds since 1Jan1904"=timestamp(3822528646.8947263 s since 1904-01-01), "mean[ps]"=46.683525649931155}, {"seconds since 1Jan1904"=timestamp(3822528948.387137 s since 1904-01-01), "mean[ps]"=46.925296519909544}, {"seconds since 1Jan1904"=timestamp(3822529249.822836 s since 1904-01-01), "mean[ps]"=48.67492747385779}, {"seconds since 1Jan1904"=timestamp(3822529551.2237015 s since 1904-01-01), "mean[ps]"=47.85580348886559}, {"seconds since 1Jan1904"=timestamp(3822529852.7132487 s since 1904-01-01), "mean[ps]"=47.020694398044704}, {"seconds since 1Jan1904"=timestamp(3822530154.13355 s since 1904-01-01), "mean[ps]"=47.174682061041295}, {"seconds since 1Jan1904"=timestamp(3822530455.5063615 s since 1904-01-01), "mean[ps]"=45.16331138598638}, {"seconds since 1Jan1904"=timestamp(3822530756.906737 s since 1904-01-01), "mean[ps]"=46.43753883169593}, {"seconds since 1Jan1904"=timestamp(3822531058.404439 s since 1904-01-01), "mean[ps]"=47.11139943016023}, {"seconds since 1Jan1904"=timestamp(3822531359.808485 s since 1904-01-01), "mean[ps]"=46.7829856150822}, {"seconds since 1Jan1904"=timestamp(3822531661.336039 s since 1904-01-01), "mean[ps]"=48.51666868420625}, {"seconds since 1Jan1904"=timestamp(3822531962.7850113 s since 1904-01-01), "mean[ps]"=48.43600403332135}, {"seconds since 1Jan1904"=timestamp(3822532264.2264094 s since 1904-01-01), "mean[ps]"=47.76467661695182}, {"seconds since 1Jan1904"=timestamp(3822532565.644325 s since 1904-01-01), "mean[ps]"=46.939606199227065}, {"seconds since 1Jan1904"=timestamp(3822532867.095218 s since 1904-01-01), "mean[ps]"=47.071507378928956}, {"seconds since 1Jan1904"=timestamp(3822533168.4954033 s since 1904-01-01), "mean[ps]"=47.431361442938545}, {"seconds since 1Jan1904"=timestamp(3822533470.0292826 s since 1904-01-01), "mean[ps]"=46.9518237402652}, {"seconds since 1Jan1904"=timestamp(3822533771.460639 s since 1904-01-01), "mean[ps]"=45.84324039161155}, {"seconds since 1Jan1904"=timestamp(3822534072.903432 s since 1904-01-01), "mean[ps]"=45.36436317284198}, {"seconds since 1Jan1904"=timestamp(3822534374.327941 s since 1904-01-01), "mean[ps]"=48.56462440228474}, {"seconds since 1Jan1904"=timestamp(3822534675.8510175 s since 1904-01-01), "mean[ps]"=48.41034097984737}, {"seconds since 1Jan1904"=timestamp(3822534977.3926754 s since 1904-01-01), "mean[ps]"=48.882181416674165}, {"seconds since 1Jan1904"=timestamp(3822535278.8113256 s since 1904-01-01), "mean[ps]"=47.65235620100664}, {"seconds since 1Jan1904"=timestamp(3822535580.052392 s since 1904-01-01), "mean[ps]"=46.96539843246671}, {"seconds since 1Jan1904"=timestamp(3822535881.6109457 s since 1904-01-01), "mean[ps]"=48.75998325048443}, {"seconds since 1Jan1904"=timestamp(3822536183.1016607 s since 1904-01-01), "mean[ps]"=48.380476076555304}, {"seconds since 1Jan1904"=timestamp(3822536484.4703193 s since 1904-01-01), "mean[ps]"=47.62115394503704}, {"seconds since 1Jan1904"=timestamp(3822536786.003652 s since 1904-01-01), "mean[ps]"=50.30766656415301}, {"seconds since 1Jan1904"=timestamp(3822537087.3877025 s since 1904-01-01), "mean[ps]"=47.48690978145481}, {"seconds since 1Jan1904"=timestamp(3822537388.9627695 s since 1904-01-01), "mean[ps]"=46.15965302647617}, {"seconds since 1Jan1904"=timestamp(3822537690.32478 s since 1904-01-01), "mean[ps]"=47.490035534119265}, {"seconds since 1Jan1904"=timestamp(3822537991.8736057 s since 1904-01-01), "mean[ps]"=46.089278009915134}, {"seconds since 1Jan1904"=timestamp(3822538293.281887 s since 1904-01-01), "mean[ps]"=47.8245829523465}, {"seconds since 1Jan1904"=timestamp(3822538594.700456 s since 1904-01-01), "mean[ps]"=49.933893516404545}, {"seconds since 1Jan1904"=timestamp(3822538896.2253175 s since 1904-01-01), "mean[ps]"=50.36985123493083}, {"seconds since 1Jan1904"=timestamp(3822539197.7020054 s since 1904-01-01), "mean[ps]"=47.17554176070486}, {"seconds since 1Jan1904"=timestamp(3822539499.1529503 s since 1904-01-01), "mean[ps]"=46.780114684027055}, {"seconds since 1Jan1904"=timestamp(3822539800.5176826 s since 1904-01-01), "mean[ps]"=47.505212661194456}, {"seconds since 1Jan1904"=timestamp(3822540101.955672 s since 1904-01-01), "mean[ps]"=44.460046111779135}, {"seconds since 1Jan1904"=timestamp(3822540403.389026 s since 1904-01-01), "mean[ps]"=46.61969388523377}, {"seconds since 1Jan1904"=timestamp(3822540704.8647823 s since 1904-01-01), "mean[ps]"=47.64016779716088}, {"seconds since 1Jan1904"=timestamp(3822541006.2905207 s since 1904-01-01), "mean[ps]"=45.87981422071646}, {"seconds since 1Jan1904"=timestamp(3822541307.8066297 s since 1904-01-01), "mean[ps]"=47.6951023861682}, {"seconds since 1Jan1904"=timestamp(3822541609.3079934 s since 1904-01-01), "mean[ps]"=48.885335535304776}, {"seconds since 1Jan1904"=timestamp(3822541910.788964 s since 1904-01-01), "mean[ps]"=48.3755223007449}, {"seconds since 1Jan1904"=timestamp(3822542212.360313 s since 1904-01-01), "mean[ps]"=46.43887572587223}, {"seconds since 1Jan1904"=timestamp(3822542513.8452806 s since 1904-01-01), "mean[ps]"=48.47816349737167}, {"seconds since 1Jan1904"=timestamp(3822542815.328869 s since 1904-01-01), "mean[ps]"=46.357280854600766}, {"seconds since 1Jan1904"=timestamp(3822543116.8031616 s since 1904-01-01), "mean[ps]"=45.547398463823825}, {"seconds since 1Jan1904"=timestamp(3822543418.253579 s since 1904-01-01), "mean[ps]"=47.226538550536524}, {"seconds since 1Jan1904"=timestamp(3822543719.8005633 s since 1904-01-01), "mean[ps]"=45.86103026572485}, {"seconds since 1Jan1904"=timestamp(3822544021.284577 s since 1904-01-01), "mean[ps]"=48.72586993708444}, {"seconds since 1Jan1904"=timestamp(3822544322.8030105 s since 1904-01-01), "mean[ps]"=47.81818366111602}, {"seconds since 1Jan1904"=timestamp(3822544624.2975945 s since 1904-01-01), "mean[ps]"=46.730725922259154}, {"seconds since 1Jan1904"=timestamp(3822544925.818383 s since 1904-01-01), "mean[ps]"=46.84779183865165}, {"seconds since 1Jan1904"=timestamp(3822545227.2305446 s since 1904-01-01), "mean[ps]"=46.53126651704602}, {"seconds since 1Jan1904"=timestamp(3822545528.6374345 s since 1904-01-01), "mean[ps]"=47.327906007280326}, {"seconds since 1Jan1904"=timestamp(3822545830.161919 s since 1904-01-01), "mean[ps]"=46.238918656078724}, {"seconds since 1Jan1904"=timestamp(3822546131.6581616 s since 1904-01-01), "mean[ps]"=47.119349645852715}, {"seconds since 1Jan1904"=timestamp(3822546433.1208367 s since 1904-01-01), "mean[ps]"=48.08876248505623}, {"seconds since 1Jan1904"=timestamp(3822546734.5235424 s since 1904-01-01), "mean[ps]"=46.71312799777554}, {"seconds since 1Jan1904"=timestamp(3822547035.9215217 s since 1904-01-01), "mean[ps]"=47.24133309665515}, {"seconds since 1Jan1904"=timestamp(3822547337.4649706 s since 1904-01-01), "mean[ps]"=46.55333135836854}, {"seconds since 1Jan1904"=timestamp(3822547638.88064 s since 1904-01-01), "mean[ps]"=46.92414715587934}, {"seconds since 1Jan1904"=timestamp(3822547940.3121905 s since 1904-01-01), "mean[ps]"=48.357955676549935}, {"seconds since 1Jan1904"=timestamp(3822548241.74978 s since 1904-01-01), "mean[ps]"=48.736959612455856}, {"seconds since 1Jan1904"=timestamp(3822548543.2799606 s since 1904-01-01), "mean[ps]"=48.04994333397735}, {"seconds since 1Jan1904"=timestamp(3822548844.742632 s since 1904-01-01), "mean[ps]"=47.06485299731205}, {"seconds since 1Jan1904"=timestamp(3822549146.149104 s since 1904-01-01), "mean[ps]"=48.01914354989339}, {"seconds since 1Jan1904"=timestamp(3822549447.533661 s since 1904-01-01), "mean[ps]"=47.67501864449972}, {"seconds since 1Jan1904"=timestamp(3822549748.9579425 s since 1904-01-01), "mean[ps]"=45.95478090138256}, {"seconds since 1Jan1904"=timestamp(3822550050.4716654 s since 1904-01-01), "mean[ps]"=47.683024702357024}, {"seconds since 1Jan1904"=timestamp(3822550351.947339 s since 1904-01-01), "mean[ps]"=47.55358632826086}, {"seconds since 1Jan1904"=timestamp(3822550653.458123 s since 1904-01-01), "mean[ps]"=46.18456934487834}, {"seconds since 1Jan1904"=timestamp(3822550954.99518 s since 1904-01-01), "mean[ps]"=47.49603026130894}, {"seconds since 1Jan1904"=timestamp(3822551256.5036974 s since 1904-01-01), "mean[ps]"=47.695201593090324}, {"seconds since 1Jan1904"=timestamp(3822551558.0137887 s since 1904-01-01), "mean[ps]"=45.87588027389053}, {"seconds since 1Jan1904"=timestamp(3822551859.5051265 s since 1904-01-01), "mean[ps]"=47.147683662639274}, {"seconds since 1Jan1904"=timestamp(3822552161.039615 s since 1904-01-01), "mean[ps]"=45.672541572570225}, {"seconds since 1Jan1904"=timestamp(3822552462.609901 s since 1904-01-01), "mean[ps]"=47.970736141807336}, {"seconds since 1Jan1904"=timestamp(3822552764.000548 s since 1904-01-01), "mean[ps]"=48.47553755949918}, {"seconds since 1Jan1904"=timestamp(3822553065.419496 s since 1904-01-01), "mean[ps]"=47.74201718437574}, {"seconds since 1Jan1904"=timestamp(3822553366.9214015 s since 1904-01-01), "mean[ps]"=47.15255927445895}, {"seconds since 1Jan1904"=timestamp(3822553668.2656054 s since 1904-01-01), "mean[ps]"=47.51164947674246}, {"seconds since 1Jan1904"=timestamp(3822553969.7844114 s since 1904-01-01), "mean[ps]"=47.19341865641025}, {"seconds since 1Jan1904"=timestamp(3822554271.2343993 s since 1904-01-01), "mean[ps]"=49.95758696058103}, {"seconds since 1Jan1904"=timestamp(3822554572.7825623 s since 1904-01-01), "mean[ps]"=46.77988961443474}, {"seconds since 1Jan1904"=timestamp(3822554874.2372446 s since 1904-01-01), "mean[ps]"=48.289835994599066}, {"seconds since 1Jan1904"=timestamp(3822555175.792369 s since 1904-01-01), "mean[ps]"=48.50385399524389}, {"seconds since 1Jan1904"=timestamp(3822555477.2372074 s since 1904-01-01), "mean[ps]"=49.629125269520046}, {"seconds since 1Jan1904"=timestamp(3822555778.701035 s since 1904-01-01), "mean[ps]"=45.43456709133414}, {"seconds since 1Jan1904"=timestamp(3822556080.2516418 s since 1904-01-01), "mean[ps]"=48.24865192968874}, {"seconds since 1Jan1904"=timestamp(3822556381.757804 s since 1904-01-01), "mean[ps]"=49.69735249467746}, {"seconds since 1Jan1904"=timestamp(3822556683.148675 s since 1904-01-01), "mean[ps]"=46.3781002697528}, {"seconds since 1Jan1904"=timestamp(3822556984.6444607 s since 1904-01-01), "mean[ps]"=45.34991853033499}, {"seconds since 1Jan1904"=timestamp(3822557286.095585 s since 1904-01-01), "mean[ps]"=45.27205511988183}, {"seconds since 1Jan1904"=timestamp(3822557587.5588975 s since 1904-01-01), "mean[ps]"=46.87772356965683}, {"seconds since 1Jan1904"=timestamp(3822557889.0395904 s since 1904-01-01), "mean[ps]"=48.7552376389635}, {"seconds since 1Jan1904"=timestamp(3822558190.4474607 s since 1904-01-01), "mean[ps]"=49.10323500133465}, {"seconds since 1Jan1904"=timestamp(3822558492.0190606 s since 1904-01-01), "mean[ps]"=46.019668954503196}, {"seconds since 1Jan1904"=timestamp(3822558793.477814 s since 1904-01-01), "mean[ps]"=46.98047449444034}, {"seconds since 1Jan1904"=timestamp(3822559094.921321 s since 1904-01-01), "mean[ps]"=47.73712579307682}, {"seconds since 1Jan1904"=timestamp(3822559396.4460673 s since 1904-01-01), "mean[ps]"=47.379155290045745}, {"seconds since 1Jan1904"=timestamp(3822559697.9183455 s since 1904-01-01), "mean[ps]"=48.28148661172769}, {"seconds since 1Jan1904"=timestamp(3822559999.3983808 s since 1904-01-01), "mean[ps]"=49.5554776933218}, {"seconds since 1Jan1904"=timestamp(3822560300.8987856 s since 1904-01-01), "mean[ps]"=49.85119484439492}, {"seconds since 1Jan1904"=timestamp(3822560602.3556256 s since 1904-01-01), "mean[ps]"=48.45401938924547}, {"seconds since 1Jan1904"=timestamp(3822560903.899011 s since 1904-01-01), "mean[ps]"=46.625626917015026}, {"seconds since 1Jan1904"=timestamp(3822561205.442392 s since 1904-01-01), "mean[ps]"=46.403798941258174}, {"seconds since 1Jan1904"=timestamp(3822561506.864459 s since 1904-01-01), "mean[ps]"=50.741603278318124}, {"seconds since 1Jan1904"=timestamp(3822561808.4265895 s since 1904-01-01), "mean[ps]"=47.278723958942294}, {"seconds since 1Jan1904"=timestamp(3822562109.9678545 s since 1904-01-01), "mean[ps]"=46.12584811390659}, {"seconds since 1Jan1904"=timestamp(3822562411.5341334 s since 1904-01-01), "mean[ps]"=48.7674328197406}, {"seconds since 1Jan1904"=timestamp(3822562712.998142 s since 1904-01-01), "mean[ps]"=44.85597708272976}, {"seconds since 1Jan1904"=timestamp(3822563014.480204 s since 1904-01-01), "mean[ps]"=48.83854210693687}, {"seconds since 1Jan1904"=timestamp(3822563315.9980226 s since 1904-01-01), "mean[ps]"=49.77693375243968}, {"seconds since 1Jan1904"=timestamp(3822563617.240683 s since 1904-01-01), "mean[ps]"=47.808134313740254}, {"seconds since 1Jan1904"=timestamp(3822563918.749057 s since 1904-01-01), "mean[ps]"=47.81256456207577}, {"seconds since 1Jan1904"=timestamp(3822564220.254855 s since 1904-01-01), "mean[ps]"=47.80822934304376}, {"seconds since 1Jan1904"=timestamp(3822564521.8313217 s since 1904-01-01), "mean[ps]"=47.14643562037576}, {"seconds since 1Jan1904"=timestamp(3822564823.2753153 s since 1904-01-01), "mean[ps]"=49.69045854744464}, {"seconds since 1Jan1904"=timestamp(3822565124.701639 s since 1904-01-01), "mean[ps]"=46.806062608206084}, {"seconds since 1Jan1904"=timestamp(3822565426.1726537 s since 1904-01-01), "mean[ps]"=47.59980270525496}, {"seconds since 1Jan1904"=timestamp(3822565727.6830926 s since 1904-01-01), "mean[ps]"=47.24338548952519}, {"seconds since 1Jan1904"=timestamp(3822566029.165819 s since 1904-01-01), "mean[ps]"=46.89964534228151}, {"seconds since 1Jan1904"=timestamp(3822566330.740963 s since 1904-01-01), "mean[ps]"=44.70262495746521}, {"seconds since 1Jan1904"=timestamp(3822566632.249509 s since 1904-01-01), "mean[ps]"=46.06625916195626}, {"seconds since 1Jan1904"=timestamp(3822566933.704676 s since 1904-01-01), "mean[ps]"=48.639752662888824}, {"seconds since 1Jan1904"=timestamp(3822567235.209213 s since 1904-01-01), "mean[ps]"=45.426435183897276}, {"seconds since 1Jan1904"=timestamp(3822567536.6946225 s since 1904-01-01), "mean[ps]"=46.610338882745374}, {"seconds since 1Jan1904"=timestamp(3822567838.169631 s since 1904-01-01), "mean[ps]"=46.490948326763124}, {"seconds since 1Jan1904"=timestamp(3822568139.6286063 s since 1904-01-01), "mean[ps]"=46.29418847102086}, {"seconds since 1Jan1904"=timestamp(3822568441.096488 s since 1904-01-01), "mean[ps]"=47.16529975076451}, {"seconds since 1Jan1904"=timestamp(3822568742.5332594 s since 1904-01-01), "mean[ps]"=46.41495673823862}, {"seconds since 1Jan1904"=timestamp(3822569044.0896015 s since 1904-01-01), "mean[ps]"=47.06395500402215}, {"seconds since 1Jan1904"=timestamp(3822569345.551961 s since 1904-01-01), "mean[ps]"=47.205943588339835}, {"seconds since 1Jan1904"=timestamp(3822569647.024821 s since 1904-01-01), "mean[ps]"=47.023610855633265}, {"seconds since 1Jan1904"=timestamp(3822569948.559713 s since 1904-01-01), "mean[ps]"=47.690836616069696}, {"seconds since 1Jan1904"=timestamp(3822570249.9499383 s since 1904-01-01), "mean[ps]"=46.866664682645215}, {"seconds since 1Jan1904"=timestamp(3822570551.4543366 s since 1904-01-01), "mean[ps]"=46.78641011079814}, {"seconds since 1Jan1904"=timestamp(3822570852.907388 s since 1904-01-01), "mean[ps]"=46.228452971687666}, {"seconds since 1Jan1904"=timestamp(3822571154.3613434 s since 1904-01-01), "mean[ps]"=47.922723715782126}, {"seconds since 1Jan1904"=timestamp(3822571455.875889 s since 1904-01-01), "mean[ps]"=47.97811855996823}, {"seconds since 1Jan1904"=timestamp(3822571757.4035335 s since 1904-01-01), "mean[ps]"=47.70177363619977}, {"seconds since 1Jan1904"=timestamp(3822572058.8738127 s since 1904-01-01), "mean[ps]"=50.98380284505595}, {"seconds since 1Jan1904"=timestamp(3822572360.3478255 s since 1904-01-01), "mean[ps]"=47.787382002222834}, {"seconds since 1Jan1904"=timestamp(3822572661.834789 s since 1904-01-01), "mean[ps]"=49.70769479641368}, {"seconds since 1Jan1904"=timestamp(3822572963.3136296 s since 1904-01-01), "mean[ps]"=48.99465334437374}, {"seconds since 1Jan1904"=timestamp(3822573264.8089194 s since 1904-01-01), "mean[ps]"=46.54994005762823}, {"seconds since 1Jan1904"=timestamp(3822573566.2905793 s since 1904-01-01), "mean[ps]"=47.719849007666895}, {"seconds since 1Jan1904"=timestamp(3822573867.753861 s since 1904-01-01), "mean[ps]"=46.87215614366724}, {"seconds since 1Jan1904"=timestamp(3822574169.3307586 s since 1904-01-01), "mean[ps]"=46.68952333554961}, {"seconds since 1Jan1904"=timestamp(3822574470.7852354 s since 1904-01-01), "mean[ps]"=47.986790766518624}, {"seconds since 1Jan1904"=timestamp(3822574772.1922865 s since 1904-01-01), "mean[ps]"=47.400617320262796}, {"seconds since 1Jan1904"=timestamp(3822575073.6485744 s since 1904-01-01), "mean[ps]"=46.53131330077983}, {"seconds since 1Jan1904"=timestamp(3822575375.0628457 s since 1904-01-01), "mean[ps]"=45.89662046937819}, {"seconds since 1Jan1904"=timestamp(3822575676.540885 s since 1904-01-01), "mean[ps]"=48.04908355085044}, {"seconds since 1Jan1904"=timestamp(3822575978.110875 s since 1904-01-01), "mean[ps]"=47.19779180874513}, {"seconds since 1Jan1904"=timestamp(3822576279.6679864 s since 1904-01-01), "mean[ps]"=46.14946309325799}, {"seconds since 1Jan1904"=timestamp(3822576581.2032743 s since 1904-01-01), "mean[ps]"=46.49579925080451}, {"seconds since 1Jan1904"=timestamp(3822576882.6405673 s since 1904-01-01), "mean[ps]"=48.77782202830812}, {"seconds since 1Jan1904"=timestamp(3822577184.1204553 s since 1904-01-01), "mean[ps]"=47.40737626405205}, {"seconds since 1Jan1904"=timestamp(3822577485.6404696 s since 1904-01-01), "mean[ps]"=45.76192927861338}, {"seconds since 1Jan1904"=timestamp(3822577787.095057 s since 1904-01-01), "mean[ps]"=46.920304156771174}, {"seconds since 1Jan1904"=timestamp(3822578088.553026 s since 1904-01-01), "mean[ps]"=47.532618115530276}, {"seconds since 1Jan1904"=timestamp(3822578390.115008 s since 1904-01-01), "mean[ps]"=45.08113194429089}, {"seconds since 1Jan1904"=timestamp(3822578691.551293 s since 1904-01-01), "mean[ps]"=47.23507725784269}, {"seconds since 1Jan1904"=timestamp(3822578992.9199705 s since 1904-01-01), "mean[ps]"=45.423703404059694}, {"seconds since 1Jan1904"=timestamp(3822579294.3933854 s since 1904-01-01), "mean[ps]"=47.39095989734955}, {"seconds since 1Jan1904"=timestamp(3822579595.918991 s since 1904-01-01), "mean[ps]"=46.92476236594837}, {"seconds since 1Jan1904"=timestamp(3822579897.4222097 s since 1904-01-01), "mean[ps]"=46.170821938038145}, {"seconds since 1Jan1904"=timestamp(3822580198.9128265 s since 1904-01-01), "mean[ps]"=47.81821367115413}, {"seconds since 1Jan1904"=timestamp(3822580500.314174 s since 1904-01-01), "mean[ps]"=47.86296174324037}, {"seconds since 1Jan1904"=timestamp(3822580801.8501215 s since 1904-01-01), "mean[ps]"=47.606239800153595}, {"seconds since 1Jan1904"=timestamp(3822581103.3778 s since 1904-01-01), "mean[ps]"=46.053949236485806}, {"seconds since 1Jan1904"=timestamp(3822581404.880745 s since 1904-01-01), "mean[ps]"=47.10746302182636}, {"seconds since 1Jan1904"=timestamp(3822581706.4360175 s since 1904-01-01), "mean[ps]"=47.53723866912824}, {"seconds since 1Jan1904"=timestamp(3822582007.8203206 s since 1904-01-01), "mean[ps]"=49.367945639663425}, {"seconds since 1Jan1904"=timestamp(3822582309.2484713 s since 1904-01-01), "mean[ps]"=44.68410614545749}, {"seconds since 1Jan1904"=timestamp(3822582610.7182074 s since 1904-01-01), "mean[ps]"=46.17850874297742}, {"seconds since 1Jan1904"=timestamp(3822582912.221481 s since 1904-01-01), "mean[ps]"=49.36953283018316}, {"seconds since 1Jan1904"=timestamp(3822583213.701206 s since 1904-01-01), "mean[ps]"=48.37737496208425}, {"seconds since 1Jan1904"=timestamp(3822583515.2400217 s since 1904-01-01), "mean[ps]"=48.244046455647094}, {"seconds since 1Jan1904"=timestamp(3822583816.7411456 s since 1904-01-01), "mean[ps]"=47.2709078159121}, {"seconds since 1Jan1904"=timestamp(3822584118.2147617 s since 1904-01-01), "mean[ps]"=46.62622511398556}, {"seconds since 1Jan1904"=timestamp(3822584419.675927 s since 1904-01-01), "mean[ps]"=47.09198009764359}, {"seconds since 1Jan1904"=timestamp(3822584721.0923023 s since 1904-01-01), "mean[ps]"=47.09885056954355}, {"seconds since 1Jan1904"=timestamp(3822585022.5496383 s since 1904-01-01), "mean[ps]"=48.27480177245531}, {"seconds since 1Jan1904"=timestamp(3822585324.043527 s since 1904-01-01), "mean[ps]"=48.51238576890493}, {"seconds since 1Jan1904"=timestamp(3822585625.471996 s since 1904-01-01), "mean[ps]"=48.12614946647828}, {"seconds since 1Jan1904"=timestamp(3822585926.8942423 s since 1904-01-01), "mean[ps]"=47.70708158597775}, {"seconds since 1Jan1904"=timestamp(3822586228.3225694 s since 1904-01-01), "mean[ps]"=48.302861400595646}, {"seconds since 1Jan1904"=timestamp(3822586529.8338766 s since 1904-01-01), "mean[ps]"=46.145496795679705}, {"seconds since 1Jan1904"=timestamp(3822586831.2920294 s since 1904-01-01), "mean[ps]"=47.821213690856936}, {"seconds since 1Jan1904"=timestamp(3822587132.7088814 s since 1904-01-01), "mean[ps]"=47.46871671227752}, {"seconds since 1Jan1904"=timestamp(3822587434.1071906 s since 1904-01-01), "mean[ps]"=50.828157572179954}, {"seconds since 1Jan1904"=timestamp(3822587735.3207207 s since 1904-01-01), "mean[ps]"=47.87308964253295}, {"seconds since 1Jan1904"=timestamp(3822588036.7855854 s since 1904-01-01), "mean[ps]"=47.324596684518866}, {"seconds since 1Jan1904"=timestamp(3822588338.3446593 s since 1904-01-01), "mean[ps]"=48.540987482422416}, {"seconds since 1Jan1904"=timestamp(3822588639.839839 s since 1904-01-01), "mean[ps]"=46.10921617460086}, {"seconds since 1Jan1904"=timestamp(3822588941.288984 s since 1904-01-01), "mean[ps]"=46.38272796352157}, {"seconds since 1Jan1904"=timestamp(3822589242.7402463 s since 1904-01-01), "mean[ps]"=46.20504077776748}, {"seconds since 1Jan1904"=timestamp(3822589544.2098656 s since 1904-01-01), "mean[ps]"=48.037071551434416}, {"seconds since 1Jan1904"=timestamp(3822589845.6971216 s since 1904-01-01), "mean[ps]"=46.856271036830464}, {"seconds since 1Jan1904"=timestamp(3822590147.2125216 s since 1904-01-01), "mean[ps]"=47.113221174266926}, {"seconds since 1Jan1904"=timestamp(3822590448.640258 s since 1904-01-01), "mean[ps]"=47.82032260025412}, {"seconds since 1Jan1904"=timestamp(3822590750.1391034 s since 1904-01-01), "mean[ps]"=47.60753196581295}, {"seconds since 1Jan1904"=timestamp(3822591051.5836415 s since 1904-01-01), "mean[ps]"=49.107213148009095}, {"seconds since 1Jan1904"=timestamp(3822591352.9831247 s since 1904-01-01), "mean[ps]"=47.563412726415464}, {"seconds since 1Jan1904"=timestamp(3822591654.485979 s since 1904-01-01), "mean[ps]"=47.15374798723124}, {"seconds since 1Jan1904"=timestamp(3822591955.859042 s since 1904-01-01), "mean[ps]"=45.40537653465094}, {"seconds since 1Jan1904"=timestamp(3822592257.408669 s since 1904-01-01), "mean[ps]"=51.40714905962563}, {"seconds since 1Jan1904"=timestamp(3822592558.932187 s since 1904-01-01), "mean[ps]"=46.76775467081113}, {"seconds since 1Jan1904"=timestamp(3822592860.391513 s since 1904-01-01), "mean[ps]"=47.41353077393142}, {"seconds since 1Jan1904"=timestamp(3822593161.860652 s since 1904-01-01), "mean[ps]"=47.74905559566618}, {"seconds since 1Jan1904"=timestamp(3822593463.385323 s since 1904-01-01), "mean[ps]"=47.56726134954354}, {"seconds since 1Jan1904"=timestamp(3822593764.8500686 s since 1904-01-01), "mean[ps]"=48.02909738334321}, {"seconds since 1Jan1904"=timestamp(3822594066.308588 s since 1904-01-01), "mean[ps]"=48.1655569123746}, {"seconds since 1Jan1904"=timestamp(3822594367.780607 s since 1904-01-01), "mean[ps]"=46.19336761725423}, {"seconds since 1Jan1904"=timestamp(3822594669.2577024 s since 1904-01-01), "mean[ps]"=49.09206746556864}, {"seconds since 1Jan1904"=timestamp(3822594970.726291 s since 1904-01-01), "mean[ps]"=45.868181898836276}, {"seconds since 1Jan1904"=timestamp(3822595272.1390114 s since 1904-01-01), "mean[ps]"=46.66647212786865}, {"seconds since 1Jan1904"=timestamp(3822595573.6779704 s since 1904-01-01), "mean[ps]"=48.35248729391724}, {"seconds since 1Jan1904"=timestamp(3822595875.2007656 s since 1904-01-01), "mean[ps]"=47.432773980039435}, {"seconds since 1Jan1904"=timestamp(3822596176.6578298 s since 1904-01-01), "mean[ps]"=46.945090495947916}, {"seconds since 1Jan1904"=timestamp(3822596478.2190976 s since 1904-01-01), "mean[ps]"=48.3166603847018}, {"seconds since 1Jan1904"=timestamp(3822596779.7422447 s since 1904-01-01), "mean[ps]"=47.672473949998285}, {"seconds since 1Jan1904"=timestamp(3822597081.1809144 s since 1904-01-01), "mean[ps]"=48.24305951574999}, {"seconds since 1Jan1904"=timestamp(3822597382.686327 s since 1904-01-01), "mean[ps]"=48.24184008787203}, {"seconds since 1Jan1904"=timestamp(3822597684.2478952 s since 1904-01-01), "mean[ps]"=46.24720828714593}, {"seconds since 1Jan1904"=timestamp(3822597985.7226458 s since 1904-01-01), "mean[ps]"=48.02330615545592}, {"seconds since 1Jan1904"=timestamp(3822598287.212348 s since 1904-01-01), "mean[ps]"=49.5861233370742}, {"seconds since 1Jan1904"=timestamp(3822598588.6026154 s since 1904-01-01), "mean[ps]"=48.092285046528275}, {"seconds since 1Jan1904"=timestamp(3822598890.0572553 s since 1904-01-01), "mean[ps]"=46.753409126126044}, {"seconds since 1Jan1904"=timestamp(3822599191.425584 s since 1904-01-01), "mean[ps]"=48.05646690939648}, {"seconds since 1Jan1904"=timestamp(3822599492.866769 s since 1904-01-01), "mean[ps]"=47.200601064009135}, {"seconds since 1Jan1904"=timestamp(3822599794.2904983 s since 1904-01-01), "mean[ps]"=45.98411949186585}, {"seconds since 1Jan1904"=timestamp(3822600095.7871695 s since 1904-01-01), "mean[ps]"=46.73254289056312}, {"seconds since 1Jan1904"=timestamp(3822600397.4508214 s since 1904-01-01), "mean[ps]"=48.12802724212655}, {"seconds since 1Jan1904"=timestamp(3822600698.83722 s since 1904-01-01), "mean[ps]"=47.345210970901164}, {"seconds since 1Jan1904"=timestamp(3822601000.21038 s since 1904-01-01), "mean[ps]"=47.06169434298715}, {"seconds since 1Jan1904"=timestamp(3822601301.7260976 s since 1904-01-01), "mean[ps]"=47.77065519923074}]
  in  "times":i32=400
  out "mean[ps]":dbl=-3054.7454932846654 format="%0.2f"
  out "seconds since 1Jan1904":timestamp=timestamp(3822601603.0946374 s since 1904-01-01)
  out "Counter":i32=314
  out "Mean":T1(graph)=[{"seconds since 1Jan1904"=timestamp(3822506942.315674 s since 1904-01-01), "mean[ps]"=-3071.079304876405}, {"seconds since 1Jan1904"=timestamp(3822507243.6711025 s since 1904-01-01), "mean[ps]"=-3062.959593329543}, {"seconds since 1Jan1904"=timestamp(3822507545.1626496 s since 1904-01-01), "mean[ps]"=-3058.8321662894823}, {"seconds since 1Jan1904"=timestamp(3822507846.553396 s since 1904-01-01), "mean[ps]"=-3057.9083323765303}, {"seconds since 1Jan1904"=timestamp(3822508148.061275 s since 1904-01-01), "mean[ps]"=-3061.240452072465}, {"seconds since 1Jan1904"=timestamp(3822508449.501727 s since 1904-01-01), "mean[ps]"=-3036.370323960676}, {"seconds since 1Jan1904"=timestamp(3822508750.8988624 s since 1904-01-01), "mean[ps]"=-3036.370241351195}, {"seconds since 1Jan1904"=timestamp(3822509052.3161006 s since 1904-01-01), "mean[ps]"=-3049.0215615252746}, {"seconds since 1Jan1904"=timestamp(3822509353.734636 s since 1904-01-01), "mean[ps]"=-3045.297143922103}, {"seconds since 1Jan1904"=timestamp(3822509655.1987686 s since 1904-01-01), "mean[ps]"=-3055.201042305207}, {"seconds since 1Jan1904"=timestamp(3822509956.4995074 s since 1904-01-01), "mean[ps]"=-3054.1353706805653}, {"seconds since 1Jan1904"=timestamp(3822510257.982245 s since 1904-01-01), "mean[ps]"=-3052.5574843410664}, {"seconds since 1Jan1904"=timestamp(3822510559.3960705 s since 1904-01-01), "mean[ps]"=-3049.0826084597825}, {"seconds since 1Jan1904"=timestamp(3822510860.7242055 s since 1904-01-01), "mean[ps]"=-3055.2304782891156}, {"seconds since 1Jan1904"=timestamp(3822511162.215253 s since 1904-01-01), "mean[ps]"=-3047.513467307733}, {"seconds since 1Jan1904"=timestamp(3822511463.639548 s since 1904-01-01), "mean[ps]"=-3048.9730229982188}, {"seconds since 1Jan1904"=timestamp(3822511765.766084 s since 1904-01-01), "mean[ps]"=-3063.022909455828}, {"seconds since 1Jan1904"=timestamp(3822512067.2562017 s since 1904-01-01), "mean[ps]"=-3055.8129576882566}, {"seconds since 1Jan1904"=timestamp(3822512368.655607 s since 1904-01-01), "mean[ps]"=-3052.398367104232}, {"seconds since 1Jan1904"=timestamp(3822512670.1464553 s since 1904-01-01), "mean[ps]"=-3051.7847976293706}, {"seconds since 1Jan1904"=timestamp(3822512971.507803 s since 1904-01-01), "mean[ps]"=-3065.158473670088}, {"seconds since 1Jan1904"=timestamp(3822513272.925895 s since 1904-01-01), "mean[ps]"=-3046.9007977817555}, {"seconds since 1Jan1904"=timestamp(3822513574.303528 s since 1904-01-01), "mean[ps]"=-3052.4076145763015}, {"seconds since 1Jan1904"=timestamp(3822513875.706833 s since 1904-01-01), "mean[ps]"=-3038.335094563064}, {"seconds since 1Jan1904"=timestamp(3822514177.255216 s since 1904-01-01), "mean[ps]"=-3055.3003377028513}, {"seconds since 1Jan1904"=timestamp(3822514478.6136312 s since 1904-01-01), "mean[ps]"=-3054.37946847742}, {"seconds since 1Jan1904"=timestamp(3822514780.1012654 s since 1904-01-01), "mean[ps]"=-3049.992071798466}, {"seconds since 1Jan1904"=timestamp(3822515081.6113095 s since 1904-01-01), "mean[ps]"=-3041.6094168417417}, {"seconds since 1Jan1904"=timestamp(3822515382.9461207 s since 1904-01-01), "mean[ps]"=-3057.343995368339}, {"seconds since 1Jan1904"=timestamp(3822515684.3828025 s since 1904-01-01), "mean[ps]"=-3056.0768514073466}, {"seconds since 1Jan1904"=timestamp(3822515985.8758097 s since 1904-01-01), "mean[ps]"=-3072.7544913900756}, {"seconds since 1Jan1904"=timestamp(3822516287.3353777 s since 1904-01-01), "mean[ps]"=-3060.631030670596}, {"seconds since 1Jan1904"=timestamp(3822516588.8038144 s since 1904-01-01), "mean[ps]"=-3050.458447583227}, {"seconds since 1Jan1904"=timestamp(3822516890.2282143 s since 1904-01-01), "mean[ps]"=-3063.8027528882594}, {"seconds since 1Jan1904"=timestamp(3822517191.6262407 s since 1904-01-01), "mean[ps]"=-3060.79201103057}, {"seconds since 1Jan1904"=timestamp(3822517493.0924606 s since 1904-01-01), "mean[ps]"=-3053.4786105971057}, {"seconds since 1Jan1904"=timestamp(3822517794.532418 s since 1904-01-01), "mean[ps]"=-3056.4449037031527}, {"seconds since 1Jan1904"=timestamp(3822518095.958946 s since 1904-01-01), "mean[ps]"=-3063.078799354165}, {"seconds since 1Jan1904"=timestamp(3822518397.3720393 s since 1904-01-01), "mean[ps]"=-3068.2428517019102}, {"seconds since 1Jan1904"=timestamp(3822518698.777503 s since 1904-01-01), "mean[ps]"=-3058.9650768660817}, {"seconds since 1Jan1904"=timestamp(3822519000.1937714 s since 1904-01-01), "mean[ps]"=-3050.9576890457524}, {"seconds since 1Jan1904"=timestamp(3822519301.6194086 s since 1904-01-01), "mean[ps]"=-3048.586220492143}, {"seconds since 1Jan1904"=timestamp(3822519603.042124 s since 1904-01-01), "mean[ps]"=-3065.323763769013}, {"seconds since 1Jan1904"=timestamp(3822519904.578883 s since 1904-01-01), "mean[ps]"=-3057.3496526240597}, {"seconds since 1Jan1904"=timestamp(3822520206.0544343 s since 1904-01-01), "mean[ps]"=-3056.8940798840918}, {"seconds since 1Jan1904"=timestamp(3822520507.509728 s since 1904-01-01), "mean[ps]"=-3061.0239185320966}, {"seconds since 1Jan1904"=timestamp(3822520809.0371656 s since 1904-01-01), "mean[ps]"=-3049.8380957195577}, {"seconds since 1Jan1904"=timestamp(3822521110.5518007 s since 1904-01-01), "mean[ps]"=-3070.808439854736}, {"seconds since 1Jan1904"=timestamp(3822521411.9820223 s since 1904-01-01), "mean[ps]"=-3060.267535950491}, {"seconds since 1Jan1904"=timestamp(3822521713.4490914 s since 1904-01-01), "mean[ps]"=-3053.003447055884}, {"seconds since 1Jan1904"=timestamp(3822522014.93792 s since 1904-01-01), "mean[ps]"=-3048.594918327095}, {"seconds since 1Jan1904"=timestamp(3822522316.3927464 s since 1904-01-01), "mean[ps]"=-3053.516400370868}, {"seconds since 1Jan1904"=timestamp(3822522617.8067694 s since 1904-01-01), "mean[ps]"=-3063.2403676959007}, {"seconds since 1Jan1904"=timestamp(3822522919.2539024 s since 1904-01-01), "mean[ps]"=-3041.353232328192}, {"seconds since 1Jan1904"=timestamp(3822523220.6865177 s since 1904-01-01), "mean[ps]"=-3046.79067839365}, {"seconds since 1Jan1904"=timestamp(3822523522.1590304 s since 1904-01-01), "mean[ps]"=-3046.1523996387505}, {"seconds since 1Jan1904"=timestamp(3822523823.5384583 s since 1904-01-01), "mean[ps]"=-3053.2642585862345}, {"seconds since 1Jan1904"=timestamp(3822524124.9813824 s since 1904-01-01), "mean[ps]"=-3060.6817451618676}, {"seconds since 1Jan1904"=timestamp(3822524426.491788 s since 1904-01-01), "mean[ps]"=-3054.3710473193896}, {"seconds since 1Jan1904"=timestamp(3822524727.9125314 s since 1904-01-01), "mean[ps]"=-3040.5518753116507}, {"seconds since 1Jan1904"=timestamp(3822525029.379265 s since 1904-01-01), "mean[ps]"=-3055.1564540200447}, {"seconds since 1Jan1904"=timestamp(3822525330.781236 s since 1904-01-01), "mean[ps]"=-3058.5866699269623}, {"seconds since 1Jan1904"=timestamp(3822525632.329557 s since 1904-01-01), "mean[ps]"=-3060.7056947246515}, {"seconds since 1Jan1904"=timestamp(3822525933.784519 s since 1904-01-01), "mean[ps]"=-3063.562714189083}, {"seconds since 1Jan1904"=timestamp(3822526235.2852225 s since 1904-01-01), "mean[ps]"=-3062.355843950157}, {"seconds since 1Jan1904"=timestamp(3822526536.779774 s since 1904-01-01), "mean[ps]"=-3064.9602099363783}, {"seconds since 1Jan1904"=timestamp(3822526838.2156734 s since 1904-01-01), "mean[ps]"=-3055.4174530641617}, {"seconds since 1Jan1904"=timestamp(3822527139.721087 s since 1904-01-01), "mean[ps]"=-3061.254179814402}, {"seconds since 1Jan1904"=timestamp(3822527441.1896977 s since 1904-01-01), "mean[ps]"=-3060.5800386878755}, {"seconds since 1Jan1904"=timestamp(3822527742.6183696 s since 1904-01-01), "mean[ps]"=-3052.133194412098}, {"seconds since 1Jan1904"=timestamp(3822528044.0890102 s since 1904-01-01), "mean[ps]"=-3056.3004366467785}, {"seconds since 1Jan1904"=timestamp(3822528345.503568 s since 1904-01-01), "mean[ps]"=-3058.081618421218}, {"seconds since 1Jan1904"=timestamp(3822528646.8947263 s since 1904-01-01), "mean[ps]"=-3049.7255735340736}, {"seconds since 1Jan1904"=timestamp(3822528948.387137 s since 1904-01-01), "mean[ps]"=-3049.321349062257}, {"seconds since 1Jan1904"=timestamp(3822529249.822836 s since 1904-01-01), "mean[ps]"=-3058.7665596997667}, {"seconds since 1Jan1904"=timestamp(3822529551.2237015 s since 1904-01-01), "mean[ps]"=-3051.7357037565134}, {"seconds since 1Jan1904"=timestamp(3822529852.7132487 s since 1904-01-01), "mean[ps]"=-3043.613604308719}, {"seconds since 1Jan1904"=timestamp(3822530154.13355 s since 1904-01-01), "mean[ps]"=-3044.7624684694574}, {"seconds since 1Jan1904"=timestamp(3822530455.5063615 s since 1904-01-01), "mean[ps]"=-3048.5866808878714}, {"seconds since 1Jan1904"=timestamp(3822530756.906737 s since 1904-01-01), "mean[ps]"=-3046.5033620476866}, {"seconds since 1Jan1904"=timestamp(3822531058.404439 s since 1904-01-01), "mean[ps]"=-3056.8091411381965}, {"seconds since 1Jan1904"=timestamp(3822531359.808485 s since 1904-01-01), "mean[ps]"=-3051.218342392336}, {"seconds since 1Jan1904"=timestamp(3822531661.336039 s since 1904-01-01), "mean[ps]"=-3038.9134319697037}, {"seconds since 1Jan1904"=timestamp(3822531962.7850113 s since 1904-01-01), "mean[ps]"=-3044.695507158624}, {"seconds since 1Jan1904"=timestamp(3822532264.2264094 s since 1904-01-01), "mean[ps]"=-3041.3360932425526}, {"seconds since 1Jan1904"=timestamp(3822532565.644325 s since 1904-01-01), "mean[ps]"=-3061.0045204168982}, {"seconds since 1Jan1904"=timestamp(3822532867.095218 s since 1904-01-01), "mean[ps]"=-3052.161159193967}, {"seconds since 1Jan1904"=timestamp(3822533168.4954033 s since 1904-01-01), "mean[ps]"=-3057.019421539332}, {"seconds since 1Jan1904"=timestamp(3822533470.0292826 s since 1904-01-01), "mean[ps]"=-3045.6887460636126}, {"seconds since 1Jan1904"=timestamp(3822533771.460639 s since 1904-01-01), "mean[ps]"=-3049.833886714446}, {"seconds since 1Jan1904"=timestamp(3822534072.903432 s since 1904-01-01), "mean[ps]"=-3039.0171140376574}, {"seconds since 1Jan1904"=timestamp(3822534374.327941 s since 1904-01-01), "mean[ps]"=-3045.0594079431035}, {"seconds since 1Jan1904"=timestamp(3822534675.8510175 s since 1904-01-01), "mean[ps]"=-3062.339305544034}, {"seconds since 1Jan1904"=timestamp(3822534977.3926754 s since 1904-01-01), "mean[ps]"=-3064.6956240837676}, {"seconds since 1Jan1904"=timestamp(3822535278.8113256 s since 1904-01-01), "mean[ps]"=-3047.0817241178192}, {"seconds since 1Jan1904"=timestamp(3822535580.052392 s since 1904-01-01), "mean[ps]"=-3051.2228426474776}, {"seconds since 1Jan1904"=timestamp(3822535881.6109457 s since 1904-01-01), "mean[ps]"=-3041.2210481637035}, {"seconds since 1Jan1904"=timestamp(3822536183.1016607 s since 1904-01-01), "mean[ps]"=-3048.808866720062}, {"seconds since 1Jan1904"=timestamp(3822536484.4703193 s since 1904-01-01), "mean[ps]"=-3042.192608712921}, {"seconds since 1Jan1904"=timestamp(3822536786.003652 s since 1904-01-01), "mean[ps]"=-3053.848894046506}, {"seconds since 1Jan1904"=timestamp(3822537087.3877025 s since 1904-01-01), "mean[ps]"=-3036.9486759416736}, {"seconds since 1Jan1904"=timestamp(3822537388.9627695 s since 1904-01-01), "mean[ps]"=-3043.3904144255052}, {"seconds since 1Jan1904"=timestamp(3822537690.32478 s since 1904-01-01), "mean[ps]"=-3058.542883252003}, {"seconds since 1Jan1904"=timestamp(3822537991.8736057 s since 1904-01-01), "mean[ps]"=-3048.138261288448}, {"seconds since 1Jan1904"=timestamp(3822538293.281887 s since 1904-01-01), "mean[ps]"=-3054.9163363811385}, {"seconds since 1Jan1904"=timestamp(3822538594.700456 s since 1904-01-01), "mean[ps]"=-3056.877794083271}, {"seconds since 1Jan1904"=timestamp(3822538896.2253175 s since 1904-01-01), "mean[ps]"=-3040.537571355617}, {"seconds since 1Jan1904"=timestamp(3822539197.7020054 s since 1904-01-01), "mean[ps]"=-3041.551246819542}, {"seconds since 1Jan1904"=timestamp(3822539499.1529503 s since 1904-01-01), "mean[ps]"=-3049.2829196269436}, {"seconds since 1Jan1904"=timestamp(3822539800.5176826 s since 1904-01-01), "mean[ps]"=-3049.706035975626}, {"seconds since 1Jan1904"=timestamp(3822540101.955672 s since 1904-01-01), "mean[ps]"=-3054.1965356453834}, {"seconds since 1Jan1904"=timestamp(3822540403.389026 s since 1904-01-01), "mean[ps]"=-3059.507604546281}, {"seconds since 1Jan1904"=timestamp(3822540704.8647823 s since 1904-01-01), "mean[ps]"=-3050.384459671308}, {"seconds since 1Jan1904"=timestamp(3822541006.2905207 s since 1904-01-01), "mean[ps]"=-3034.6413911904874}, {"seconds since 1Jan1904"=timestamp(3822541307.8066297 s since 1904-01-01), "mean[ps]"=-3047.7671633155633}, {"seconds since 1Jan1904"=timestamp(3822541609.3079934 s since 1904-01-01), "mean[ps]"=-3055.87670785085}, {"seconds since 1Jan1904"=timestamp(3822541910.788964 s since 1904-01-01), "mean[ps]"=-3045.9472321523585}, {"seconds since 1Jan1904"=timestamp(3822542212.360313 s since 1904-01-01), "mean[ps]"=-3054.4526312712683}, {"seconds since 1Jan1904"=timestamp(3822542513.8452806 s since 1904-01-01), "mean[ps]"=-3054.617228899252}, {"seconds since 1Jan1904"=timestamp(3822542815.328869 s since 1904-01-01), "mean[ps]"=-3062.021286641757}, {"seconds since 1Jan1904"=timestamp(3822543116.8031616 s since 1904-01-01), "mean[ps]"=-3045.108458651901}, {"seconds since 1Jan1904"=timestamp(3822543418.253579 s since 1904-01-01), "mean[ps]"=-3041.305184681364}, {"seconds since 1Jan1904"=timestamp(3822543719.8005633 s since 1904-01-01), "mean[ps]"=-3047.5227014441853}, {"seconds since 1Jan1904"=timestamp(3822544021.284577 s since 1904-01-01), "mean[ps]"=-3055.913301826102}, {"seconds since 1Jan1904"=timestamp(3822544322.8030105 s since 1904-01-01), "mean[ps]"=-3050.305149136308}, {"seconds since 1Jan1904"=timestamp(3822544624.2975945 s since 1904-01-01), "mean[ps]"=-3049.1721987887377}, {"seconds since 1Jan1904"=timestamp(3822544925.818383 s since 1904-01-01), "mean[ps]"=-3053.295992864332}, {"seconds since 1Jan1904"=timestamp(3822545227.2305446 s since 1904-01-01), "mean[ps]"=-3053.2158711978173}, {"seconds since 1Jan1904"=timestamp(3822545528.6374345 s since 1904-01-01), "mean[ps]"=-3048.707393736107}, {"seconds since 1Jan1904"=timestamp(3822545830.161919 s since 1904-01-01), "mean[ps]"=-3056.666636094031}, {"seconds since 1Jan1904"=timestamp(3822546131.6581616 s since 1904-01-01), "mean[ps]"=-3054.3244730824254}, {"seconds since 1Jan1904"=timestamp(3822546433.1208367 s since 1904-01-01), "mean[ps]"=-3050.0384260696433}, {"seconds since 1Jan1904"=timestamp(3822546734.5235424 s since 1904-01-01), "mean[ps]"=-3060.1484191595637}, {"seconds since 1Jan1904"=timestamp(3822547035.9215217 s since 1904-01-01), "mean[ps]"=-3039.4493736050304}, {"seconds since 1Jan1904"=timestamp(3822547337.4649706 s since 1904-01-01), "mean[ps]"=-3042.3614889911414}, {"seconds since 1Jan1904"=timestamp(3822547638.88064 s since 1904-01-01), "mean[ps]"=-3042.9782832199744}, {"seconds since 1Jan1904"=timestamp(3822547940.3121905 s since 1904-01-01), "mean[ps]"=-3037.6474635780824}, {"seconds since 1Jan1904"=timestamp(3822548241.74978 s since 1904-01-01), "mean[ps]"=-3042.7899903787593}, {"seconds since 1Jan1904"=timestamp(3822548543.2799606 s since 1904-01-01), "mean[ps]"=-3060.399454234211}, {"seconds since 1Jan1904"=timestamp(3822548844.742632 s since 1904-01-01), "mean[ps]"=-3051.257948203281}, {"seconds since 1Jan1904"=timestamp(3822549146.149104 s since 1904-01-01), "mean[ps]"=-3044.5002885232507}, {"seconds since 1Jan1904"=timestamp(3822549447.533661 s since 1904-01-01), "mean[ps]"=-3057.297219998728}, {"seconds since 1Jan1904"=timestamp(3822549748.9579425 s since 1904-01-01), "mean[ps]"=-3051.0292192516426}, {"seconds since 1Jan1904"=timestamp(3822550050.4716654 s since 1904-01-01), "mean[ps]"=-3040.9324410623985}, {"seconds since 1Jan1904"=timestamp(3822550351.947339 s since 1904-01-01), "mean[ps]"=-3044.5312539198558}, {"seconds since 1Jan1904"=timestamp(3822550653.458123 s since 1904-01-01), "mean[ps]"=-3056.259434771391}, {"seconds since 1Jan1904"=timestamp(3822550954.99518 s since 1904-01-01), "mean[ps]"=-3047.1194427673477}, {"seconds since 1Jan1904"=timestamp(3822551256.5036974 s since 1904-01-01), "mean[ps]"=-3037.895385842054}, {"seconds since 1Jan1904"=timestamp(3822551558.0137887 s since 1904-01-01), "mean[ps]"=-3038.4423824271717}, {"seconds since 1Jan1904"=timestamp(3822551859.5051265 s since 1904-01-01), "mean[ps]"=-3046.9785423915146}, {"seconds since 1Jan1904"=timestamp(3822552161.039615 s since 1904-01-01), "mean[ps]"=-3059.101997329547}, {"seconds since 1Jan1904"=timestamp(3822552462.609901 s since 1904-01-01), "mean[ps]"=-3045.6009752596037}, {"seconds since 1Jan1904"=timestamp(3822552764.000548 s since 1904-01-01), "mean[ps]"=-3045.0788870267834}, {"seconds since 1Jan1904"=timestamp(3822553065.419496 s since 1904-01-01), "mean[ps]"=-3051.7111572576346}, {"seconds since 1Jan1904"=timestamp(3822553366.9214015 s since 1904-01-01), "mean[ps]"=-3044.2407634979977}, {"seconds since 1Jan1904"=timestamp(3822553668.2656054 s since 1904-01-01), "mean[ps]"=-3047.0794385259123}, {"seconds since 1Jan1904"=timestamp(3822553969.7844114 s since 1904-01-01), "mean[ps]"=-3050.099971349851}, {"seconds since 1Jan1904"=timestamp(3822554271.2343993 s since 1904-01-01), "mean[ps]"=-3052.78839003927}, {"seconds since 1Jan1904"=timestamp(3822554572.7825623 s since 1904-01-01), "mean[ps]"=-3037.8444676554172}, {"seconds since 1Jan1904"=timestamp(3822554874.2372446 s since 1904-01-01), "mean[ps]"=-3045.0691799633637}, {"seconds since 1Jan1904"=timestamp(3822555175.792369 s since 1904-01-01), "mean[ps]"=-3047.8236573266213}, {"seconds since 1Jan1904"=timestamp(3822555477.2372074 s since 1904-01-01), "mean[ps]"=-3032.7814501756716}, {"seconds since 1Jan1904"=timestamp(3822555778.701035 s since 1904-01-01), "mean[ps]"=-3041.967609117142}, {"seconds since 1Jan1904"=timestamp(3822556080.2516418 s since 1904-01-01), "mean[ps]"=-3051.867060265691}, {"seconds since 1Jan1904"=timestamp(3822556381.757804 s since 1904-01-01), "mean[ps]"=-3045.494428022694}, {"seconds since 1Jan1904"=timestamp(3822556683.148675 s since 1904-01-01), "mean[ps]"=-3041.837236857799}, {"seconds since 1Jan1904"=timestamp(3822556984.6444607 s since 1904-01-01), "mean[ps]"=-3036.5973886823394}, {"seconds since 1Jan1904"=timestamp(3822557286.095585 s since 1904-01-01), "mean[ps]"=-3046.612967757018}, {"seconds since 1Jan1904"=timestamp(3822557587.5588975 s since 1904-01-01), "mean[ps]"=-3047.3506989812336}, {"seconds since 1Jan1904"=timestamp(3822557889.0395904 s since 1904-01-01), "mean[ps]"=-3037.4415254318565}, {"seconds since 1Jan1904"=timestamp(3822558190.4474607 s since 1904-01-01), "mean[ps]"=-3036.3662477926196}, {"seconds since 1Jan1904"=timestamp(3822558492.0190606 s since 1904-01-01), "mean[ps]"=-3045.526566876865}, {"seconds since 1Jan1904"=timestamp(3822558793.477814 s since 1904-01-01), "mean[ps]"=-3047.072871387049}, {"seconds since 1Jan1904"=timestamp(3822559094.921321 s since 1904-01-01), "mean[ps]"=-3052.774139713719}, {"seconds since 1Jan1904"=timestamp(3822559396.4460673 s since 1904-01-01), "mean[ps]"=-3044.2293496369393}, {"seconds since 1Jan1904"=timestamp(3822559697.9183455 s since 1904-01-01), "mean[ps]"=-3042.029550122596}, {"seconds since 1Jan1904"=timestamp(3822559999.3983808 s since 1904-01-01), "mean[ps]"=-3051.5166289243152}, {"seconds since 1Jan1904"=timestamp(3822560300.8987856 s since 1904-01-01), "mean[ps]"=-3053.168505504984}, {"seconds since 1Jan1904"=timestamp(3822560602.3556256 s since 1904-01-01), "mean[ps]"=-3032.2562062119714}, {"seconds since 1Jan1904"=timestamp(3822560903.899011 s since 1904-01-01), "mean[ps]"=-3041.764977038593}, {"seconds since 1Jan1904"=timestamp(3822561205.442392 s since 1904-01-01), "mean[ps]"=-3046.889118200257}, {"seconds since 1Jan1904"=timestamp(3822561506.864459 s since 1904-01-01), "mean[ps]"=-3050.663923125291}, {"seconds since 1Jan1904"=timestamp(3822561808.4265895 s since 1904-01-01), "mean[ps]"=-3041.109818485417}, {"seconds since 1Jan1904"=timestamp(3822562109.9678545 s since 1904-01-01), "mean[ps]"=-3041.525338192474}, {"seconds since 1Jan1904"=timestamp(3822562411.5341334 s since 1904-01-01), "mean[ps]"=-3040.7791841818976}, {"seconds since 1Jan1904"=timestamp(3822562712.998142 s since 1904-01-01), "mean[ps]"=-3045.075631099848}, {"seconds since 1Jan1904"=timestamp(3822563014.480204 s since 1904-01-01), "mean[ps]"=-3046.09498765918}, {"seconds since 1Jan1904"=timestamp(3822563315.9980226 s since 1904-01-01), "mean[ps]"=-3050.6950156078465}, {"seconds since 1Jan1904"=timestamp(3822563617.240683 s since 1904-01-01), "mean[ps]"=-3046.0651147817584}, {"seconds since 1Jan1904"=timestamp(3822563918.749057 s since 1904-01-01), "mean[ps]"=-3050.2318564294765}, {"seconds since 1Jan1904"=timestamp(3822564220.254855 s since 1904-01-01), "mean[ps]"=-3050.9777958332043}, {"seconds since 1Jan1904"=timestamp(3822564521.8313217 s since 1904-01-01), "mean[ps]"=-3047.4588890127334}, {"seconds since 1Jan1904"=timestamp(3822564823.2753153 s since 1904-01-01), "mean[ps]"=-3031.932991755758}, {"seconds since 1Jan1904"=timestamp(3822565124.701639 s since 1904-01-01), "mean[ps]"=-3047.195256207528}, {"seconds since 1Jan1904"=timestamp(3822565426.1726537 s since 1904-01-01), "mean[ps]"=-3041.818904252549}, {"seconds since 1Jan1904"=timestamp(3822565727.6830926 s since 1904-01-01), "mean[ps]"=-3036.1885514519035}, {"seconds since 1Jan1904"=timestamp(3822566029.165819 s since 1904-01-01), "mean[ps]"=-3041.3294453370117}, {"seconds since 1Jan1904"=timestamp(3822566330.740963 s since 1904-01-01), "mean[ps]"=-3027.914752816098}, {"seconds since 1Jan1904"=timestamp(3822566632.249509 s since 1904-01-01), "mean[ps]"=-3035.9520694943853}, {"seconds since 1Jan1904"=timestamp(3822566933.704676 s since 1904-01-01), "mean[ps]"=-3045.495722432267}, {"seconds since 1Jan1904"=timestamp(3822567235.209213 s since 1904-01-01), "mean[ps]"=-3042.8632008790637}, {"seconds since 1Jan1904"=timestamp(3822567536.6946225 s since 1904-01-01), "mean[ps]"=-3043.9280499573365}, {"seconds since 1Jan1904"=timestamp(3822567838.169631 s since 1904-01-01), "mean[ps]"=-3045.015089426454}, {"seconds since 1Jan1904"=timestamp(3822568139.6286063 s since 1904-01-01), "mean[ps]"=-3040.9077552078643}, {"seconds since 1Jan1904"=timestamp(3822568441.096488 s since 1904-01-01), "mean[ps]"=-3044.6502030022184}, {"seconds since 1Jan1904"=timestamp(3822568742.5332594 s since 1904-01-01), "mean[ps]"=-3038.961829880873}, {"seconds since 1Jan1904"=timestamp(3822569044.0896015 s since 1904-01-01), "mean[ps]"=-3027.6805996213766}, {"seconds since 1Jan1904"=timestamp(3822569345.551961 s since 1904-01-01), "mean[ps]"=-3057.6109015998745}, {"seconds since 1Jan1904"=timestamp(3822569647.024821 s since 1904-01-01), "mean[ps]"=-3037.0781112835525}, {"seconds since 1Jan1904"=timestamp(3822569948.559713 s since 1904-01-01), "mean[ps]"=-3049.2794051854994}, {"seconds since 1Jan1904"=timestamp(3822570249.9499383 s since 1904-01-01), "mean[ps]"=-3038.969855551546}, {"seconds since 1Jan1904"=timestamp(3822570551.4543366 s since 1904-01-01), "mean[ps]"=-3059.930672592715}, {"seconds since 1Jan1904"=timestamp(3822570852.907388 s since 1904-01-01), "mean[ps]"=-3055.8114393781602}, {"seconds since 1Jan1904"=timestamp(3822571154.3613434 s since 1904-01-01), "mean[ps]"=-3051.6480704113756}, {"seconds since 1Jan1904"=timestamp(3822571455.875889 s since 1904-01-01), "mean[ps]"=-3056.20822880477}, {"seconds since 1Jan1904"=timestamp(3822571757.4035335 s since 1904-01-01), "mean[ps]"=-3042.975429620598}, {"seconds since 1Jan1904"=timestamp(3822572058.8738127 s since 1904-01-01), "mean[ps]"=-3050.8364280372166}, {"seconds since 1Jan1904"=timestamp(3822572360.3478255 s since 1904-01-01), "mean[ps]"=-3051.1784226321925}, {"seconds since 1Jan1904"=timestamp(3822572661.834789 s since 1904-01-01), "mean[ps]"=-3044.612286328105}, {"seconds since 1Jan1904"=timestamp(3822572963.3136296 s since 1904-01-01), "mean[ps]"=-3041.552727335779}, {"seconds since 1Jan1904"=timestamp(3822573264.8089194 s since 1904-01-01), "mean[ps]"=-3039.194811846745}, {"seconds since 1Jan1904"=timestamp(3822573566.2905793 s since 1904-01-01), "mean[ps]"=-3043.198556562968}, {"seconds since 1Jan1904"=timestamp(3822573867.753861 s since 1904-01-01), "mean[ps]"=-3046.7902636713648}, {"seconds since 1Jan1904"=timestamp(3822574169.3307586 s since 1904-01-01), "mean[ps]"=-3042.394548352027}, {"seconds since 1Jan1904"=timestamp(3822574470.7852354 s since 1904-01-01), "mean[ps]"=-3046.5277622533795}, {"seconds since 1Jan1904"=timestamp(3822574772.1922865 s since 1904-01-01), "mean[ps]"=-3042.4235775326974}, {"seconds since 1Jan1904"=timestamp(3822575073.6485744 s since 1904-01-01), "mean[ps]"=-3048.90370151552}, {"seconds since 1Jan1904"=timestamp(3822575375.0628457 s since 1904-01-01), "mean[ps]"=-3037.058448870983}, {"seconds since 1Jan1904"=timestamp(3822575676.540885 s since 1904-01-01), "mean[ps]"=-3058.003893667296}, {"seconds since 1Jan1904"=timestamp(3822575978.110875 s since 1904-01-01), "mean[ps]"=-3048.038412068402}, {"seconds since 1Jan1904"=timestamp(3822576279.6679864 s since 1904-01-01), "mean[ps]"=-3057.6276981236556}, {"seconds since 1Jan1904"=timestamp(3822576581.2032743 s since 1904-01-01), "mean[ps]"=-3058.3413775233926}, {"seconds since 1Jan1904"=timestamp(3822576882.6405673 s since 1904-01-01), "mean[ps]"=-3052.7515740344043}, {"seconds since 1Jan1904"=timestamp(3822577184.1204553 s since 1904-01-01), "mean[ps]"=-3048.183111602765}, {"seconds since 1Jan1904"=timestamp(3822577485.6404696 s since 1904-01-01), "mean[ps]"=-3044.282208797018}, {"seconds since 1Jan1904"=timestamp(3822577787.095057 s since 1904-01-01), "mean[ps]"=-3057.524118137389}, {"seconds since 1Jan1904"=timestamp(3822578088.553026 s since 1904-01-01), "mean[ps]"=-3045.498094951922}, {"seconds since 1Jan1904"=timestamp(3822578390.115008 s since 1904-01-01), "mean[ps]"=-3058.524853790226}, {"seconds since 1Jan1904"=timestamp(3822578691.551293 s since 1904-01-01), "mean[ps]"=-3051.5732018566823}, {"seconds since 1Jan1904"=timestamp(3822578992.9199705 s since 1904-01-01), "mean[ps]"=-3049.562119511029}, {"seconds since 1Jan1904"=timestamp(3822579294.3933854 s since 1904-01-01), "mean[ps]"=-3054.444967087165}, {"seconds since 1Jan1904"=timestamp(3822579595.918991 s since 1904-01-01), "mean[ps]"=-3049.6331907957947}, {"seconds since 1Jan1904"=timestamp(3822579897.4222097 s since 1904-01-01), "mean[ps]"=-3046.374963244809}, {"seconds since 1Jan1904"=timestamp(3822580198.9128265 s since 1904-01-01), "mean[ps]"=-3051.0354298474886}, {"seconds since 1Jan1904"=timestamp(3822580500.314174 s since 1904-01-01), "mean[ps]"=-3055.594574447812}, {"seconds since 1Jan1904"=timestamp(3822580801.8501215 s since 1904-01-01), "mean[ps]"=-3051.453975819133}, {"seconds since 1Jan1904"=timestamp(3822581103.3778 s since 1904-01-01), "mean[ps]"=-3038.9083839669656}, {"seconds since 1Jan1904"=timestamp(3822581404.880745 s since 1904-01-01), "mean[ps]"=-3037.8028412989474}, {"seconds since 1Jan1904"=timestamp(3822581706.4360175 s since 1904-01-01), "mean[ps]"=-3051.3550994477077}, {"seconds since 1Jan1904"=timestamp(3822582007.8203206 s since 1904-01-01), "mean[ps]"=-3049.534048036431}, {"seconds since 1Jan1904"=timestamp(3822582309.2484713 s since 1904-01-01), "mean[ps]"=-3050.0068857863416}, {"seconds since 1Jan1904"=timestamp(3822582610.7182074 s since 1904-01-01), "mean[ps]"=-3035.7294854011525}, {"seconds since 1Jan1904"=timestamp(3822582912.221481 s since 1904-01-01), "mean[ps]"=-3036.976047806946}, {"seconds since 1Jan1904"=timestamp(3822583213.701206 s since 1904-01-01), "mean[ps]"=-3053.2045302696797}, {"seconds since 1Jan1904"=timestamp(3822583515.2400217 s since 1904-01-01), "mean[ps]"=-3044.2270306803016}, {"seconds since 1Jan1904"=timestamp(3822583816.7411456 s since 1904-01-01), "mean[ps]"=-3048.063495663545}, {"seconds since 1Jan1904"=timestamp(3822584118.2147617 s since 1904-01-01), "mean[ps]"=-3044.594586967812}, {"seconds since 1Jan1904"=timestamp(3822584419.675927 s since 1904-01-01), "mean[ps]"=-3045.101617033137}, {"seconds since 1Jan1904"=timestamp(3822584721.0923023 s since 1904-01-01), "mean[ps]"=-3032.950384392621}, {"seconds since 1Jan1904"=timestamp(3822585022.5496383 s since 1904-01-01), "mean[ps]"=-3036.627848109856}, {"seconds since 1Jan1904"=timestamp(3822585324.043527 s since 1904-01-01), "mean[ps]"=-3040.642753258643}, {"seconds since 1Jan1904"=timestamp(3822585625.471996 s since 1904-01-01), "mean[ps]"=-3026.6219643225527}, {"seconds since 1Jan1904"=timestamp(3822585926.8942423 s since 1904-01-01), "mean[ps]"=-3036.8850243906613}, {"seconds since 1Jan1904"=timestamp(3822586228.3225694 s since 1904-01-01), "mean[ps]"=-3042.0398240888558}, {"seconds since 1Jan1904"=timestamp(3822586529.8338766 s since 1904-01-01), "mean[ps]"=-3036.971723357878}, {"seconds since 1Jan1904"=timestamp(3822586831.2920294 s since 1904-01-01), "mean[ps]"=-3051.0958541977984}, {"seconds since 1Jan1904"=timestamp(3822587132.7088814 s since 1904-01-01), "mean[ps]"=-3040.92648783755}, {"seconds since 1Jan1904"=timestamp(3822587434.1071906 s since 1904-01-01), "mean[ps]"=-3050.1960499808642}, {"seconds since 1Jan1904"=timestamp(3822587735.3207207 s since 1904-01-01), "mean[ps]"=-3044.9681850409647}, {"seconds since 1Jan1904"=timestamp(3822588036.7855854 s since 1904-01-01), "mean[ps]"=-3048.1321382104047}, {"seconds since 1Jan1904"=timestamp(3822588338.3446593 s since 1904-01-01), "mean[ps]"=-3053.9364992403384}, {"seconds since 1Jan1904"=timestamp(3822588639.839839 s since 1904-01-01), "mean[ps]"=-3050.9769118140025}, {"seconds since 1Jan1904"=timestamp(3822588941.288984 s since 1904-01-01), "mean[ps]"=-3039.9257324358705}, {"seconds since 1Jan1904"=timestamp(3822589242.7402463 s since 1904-01-01), "mean[ps]"=-3048.496444281286}, {"seconds since 1Jan1904"=timestamp(3822589544.2098656 s since 1904-01-01), "mean[ps]"=-3043.556677447979}, {"seconds since 1Jan1904"=timestamp(3822589845.6971216 s since 1904-01-01), "mean[ps]"=-3054.9877459668746}, {"seconds since 1Jan1904"=timestamp(3822590147.2125216 s since 1904-01-01), "mean[ps]"=-3056.6682801352945}, {"seconds since 1Jan1904"=timestamp(3822590448.640258 s since 1904-01-01), "mean[ps]"=-3053.903806181417}, {"seconds since 1Jan1904"=timestamp(3822590750.1391034 s since 1904-01-01), "mean[ps]"=-3048.0680015874877}, {"seconds since 1Jan1904"=timestamp(3822591051.5836415 s since 1904-01-01), "mean[ps]"=-3063.2026348636964}, {"seconds since 1Jan1904"=timestamp(3822591352.9831247 s since 1904-01-01), "mean[ps]"=-3054.6113583404854}, {"seconds since 1Jan1904"=timestamp(3822591654.485979 s since 1904-01-01), "mean[ps]"=-3051.2042536821764}, {"seconds since 1Jan1904"=timestamp(3822591955.859042 s since 1904-01-01), "mean[ps]"=-3049.950650883677}, {"seconds since 1Jan1904"=timestamp(3822592257.408669 s since 1904-01-01), "mean[ps]"=-3052.636790609538}, {"seconds since 1Jan1904"=timestamp(3822592558.932187 s since 1904-01-01), "mean[ps]"=-3046.7852007429824}, {"seconds since 1Jan1904"=timestamp(3822592860.391513 s since 1904-01-01), "mean[ps]"=-3045.2048319990317}, {"seconds since 1Jan1904"=timestamp(3822593161.860652 s since 1904-01-01), "mean[ps]"=-3050.6248543528604}, {"seconds since 1Jan1904"=timestamp(3822593463.385323 s since 1904-01-01), "mean[ps]"=-3041.6162665691095}, {"seconds since 1Jan1904"=timestamp(3822593764.8500686 s since 1904-01-01), "mean[ps]"=-3041.0573370178568}, {"seconds since 1Jan1904"=timestamp(3822594066.308588 s since 1904-01-01), "mean[ps]"=-3039.231733164561}, {"seconds since 1Jan1904"=timestamp(3822594367.780607 s since 1904-01-01), "mean[ps]"=-3051.8764850166945}, {"seconds since 1Jan1904"=timestamp(3822594669.2577024 s since 1904-01-01), "mean[ps]"=-3044.704891352571}, {"seconds since 1Jan1904"=timestamp(3822594970.726291 s since 1904-01-01), "mean[ps]"=-3042.1702037167393}, {"seconds since 1Jan1904"=timestamp(3822595272.1390114 s since 1904-01-01), "mean[ps]"=-3039.380103230834}, {"seconds since 1Jan1904"=timestamp(3822595573.6779704 s since 1904-01-01), "mean[ps]"=-3042.632915714006}, {"seconds since 1Jan1904"=timestamp(3822595875.2007656 s since 1904-01-01), "mean[ps]"=-3050.92461002787}, {"seconds since 1Jan1904"=timestamp(3822596176.6578298 s since 1904-01-01), "mean[ps]"=-3043.7346932394453}, {"seconds since 1Jan1904"=timestamp(3822596478.2190976 s since 1904-01-01), "mean[ps]"=-3051.172655719313}, {"seconds since 1Jan1904"=timestamp(3822596779.7422447 s since 1904-01-01), "mean[ps]"=-3050.013311348962}, {"seconds since 1Jan1904"=timestamp(3822597081.1809144 s since 1904-01-01), "mean[ps]"=-3041.411720081433}, {"seconds since 1Jan1904"=timestamp(3822597382.686327 s since 1904-01-01), "mean[ps]"=-3038.4422372724807}, {"seconds since 1Jan1904"=timestamp(3822597684.2478952 s since 1904-01-01), "mean[ps]"=-3031.993174613046}, {"seconds since 1Jan1904"=timestamp(3822597985.7226458 s since 1904-01-01), "mean[ps]"=-3033.66293817821}, {"seconds since 1Jan1904"=timestamp(3822598287.212348 s since 1904-01-01), "mean[ps]"=-3056.9625638080643}, {"seconds since 1Jan1904"=timestamp(3822598588.6026154 s since 1904-01-01), "mean[ps]"=-3043.341743678329}, {"seconds since 1Jan1904"=timestamp(3822598890.0572553 s since 1904-01-01), "mean[ps]"=-3039.234635382442}, {"seconds since 1Jan1904"=timestamp(3822599191.425584 s since 1904-01-01), "mean[ps]"=-3052.403148114988}, {"seconds since 1Jan1904"=timestamp(3822599492.866769 s since 1904-01-01), "mean[ps]"=-3042.1871231085934}, {"seconds since 1Jan1904"=timestamp(3822599794.2904983 s since 1904-01-01), "mean[ps]"=-3048.553549368767}, {"seconds since 1Jan1904"=timestamp(3822600095.7871695 s since 1904-01-01), "mean[ps]"=-3053.336897273876}, {"seconds since 1Jan1904"=timestamp(3822600397.4508214 s since 1904-01-01), "mean[ps]"=-3062.5124827559684}, {"seconds since 1Jan1904"=timestamp(3822600698.83722 s since 1904-01-01), "mean[ps]"=-3058.4914785512524}, {"seconds since 1Jan1904"=timestamp(3822601000.21038 s since 1904-01-01), "mean[ps]"=-3058.654695339395}, {"seconds since 1Jan1904"=timestamp(3822601301.7260976 s since 1904-01-01), "mean[ps]"=-3054.7454932846654}]
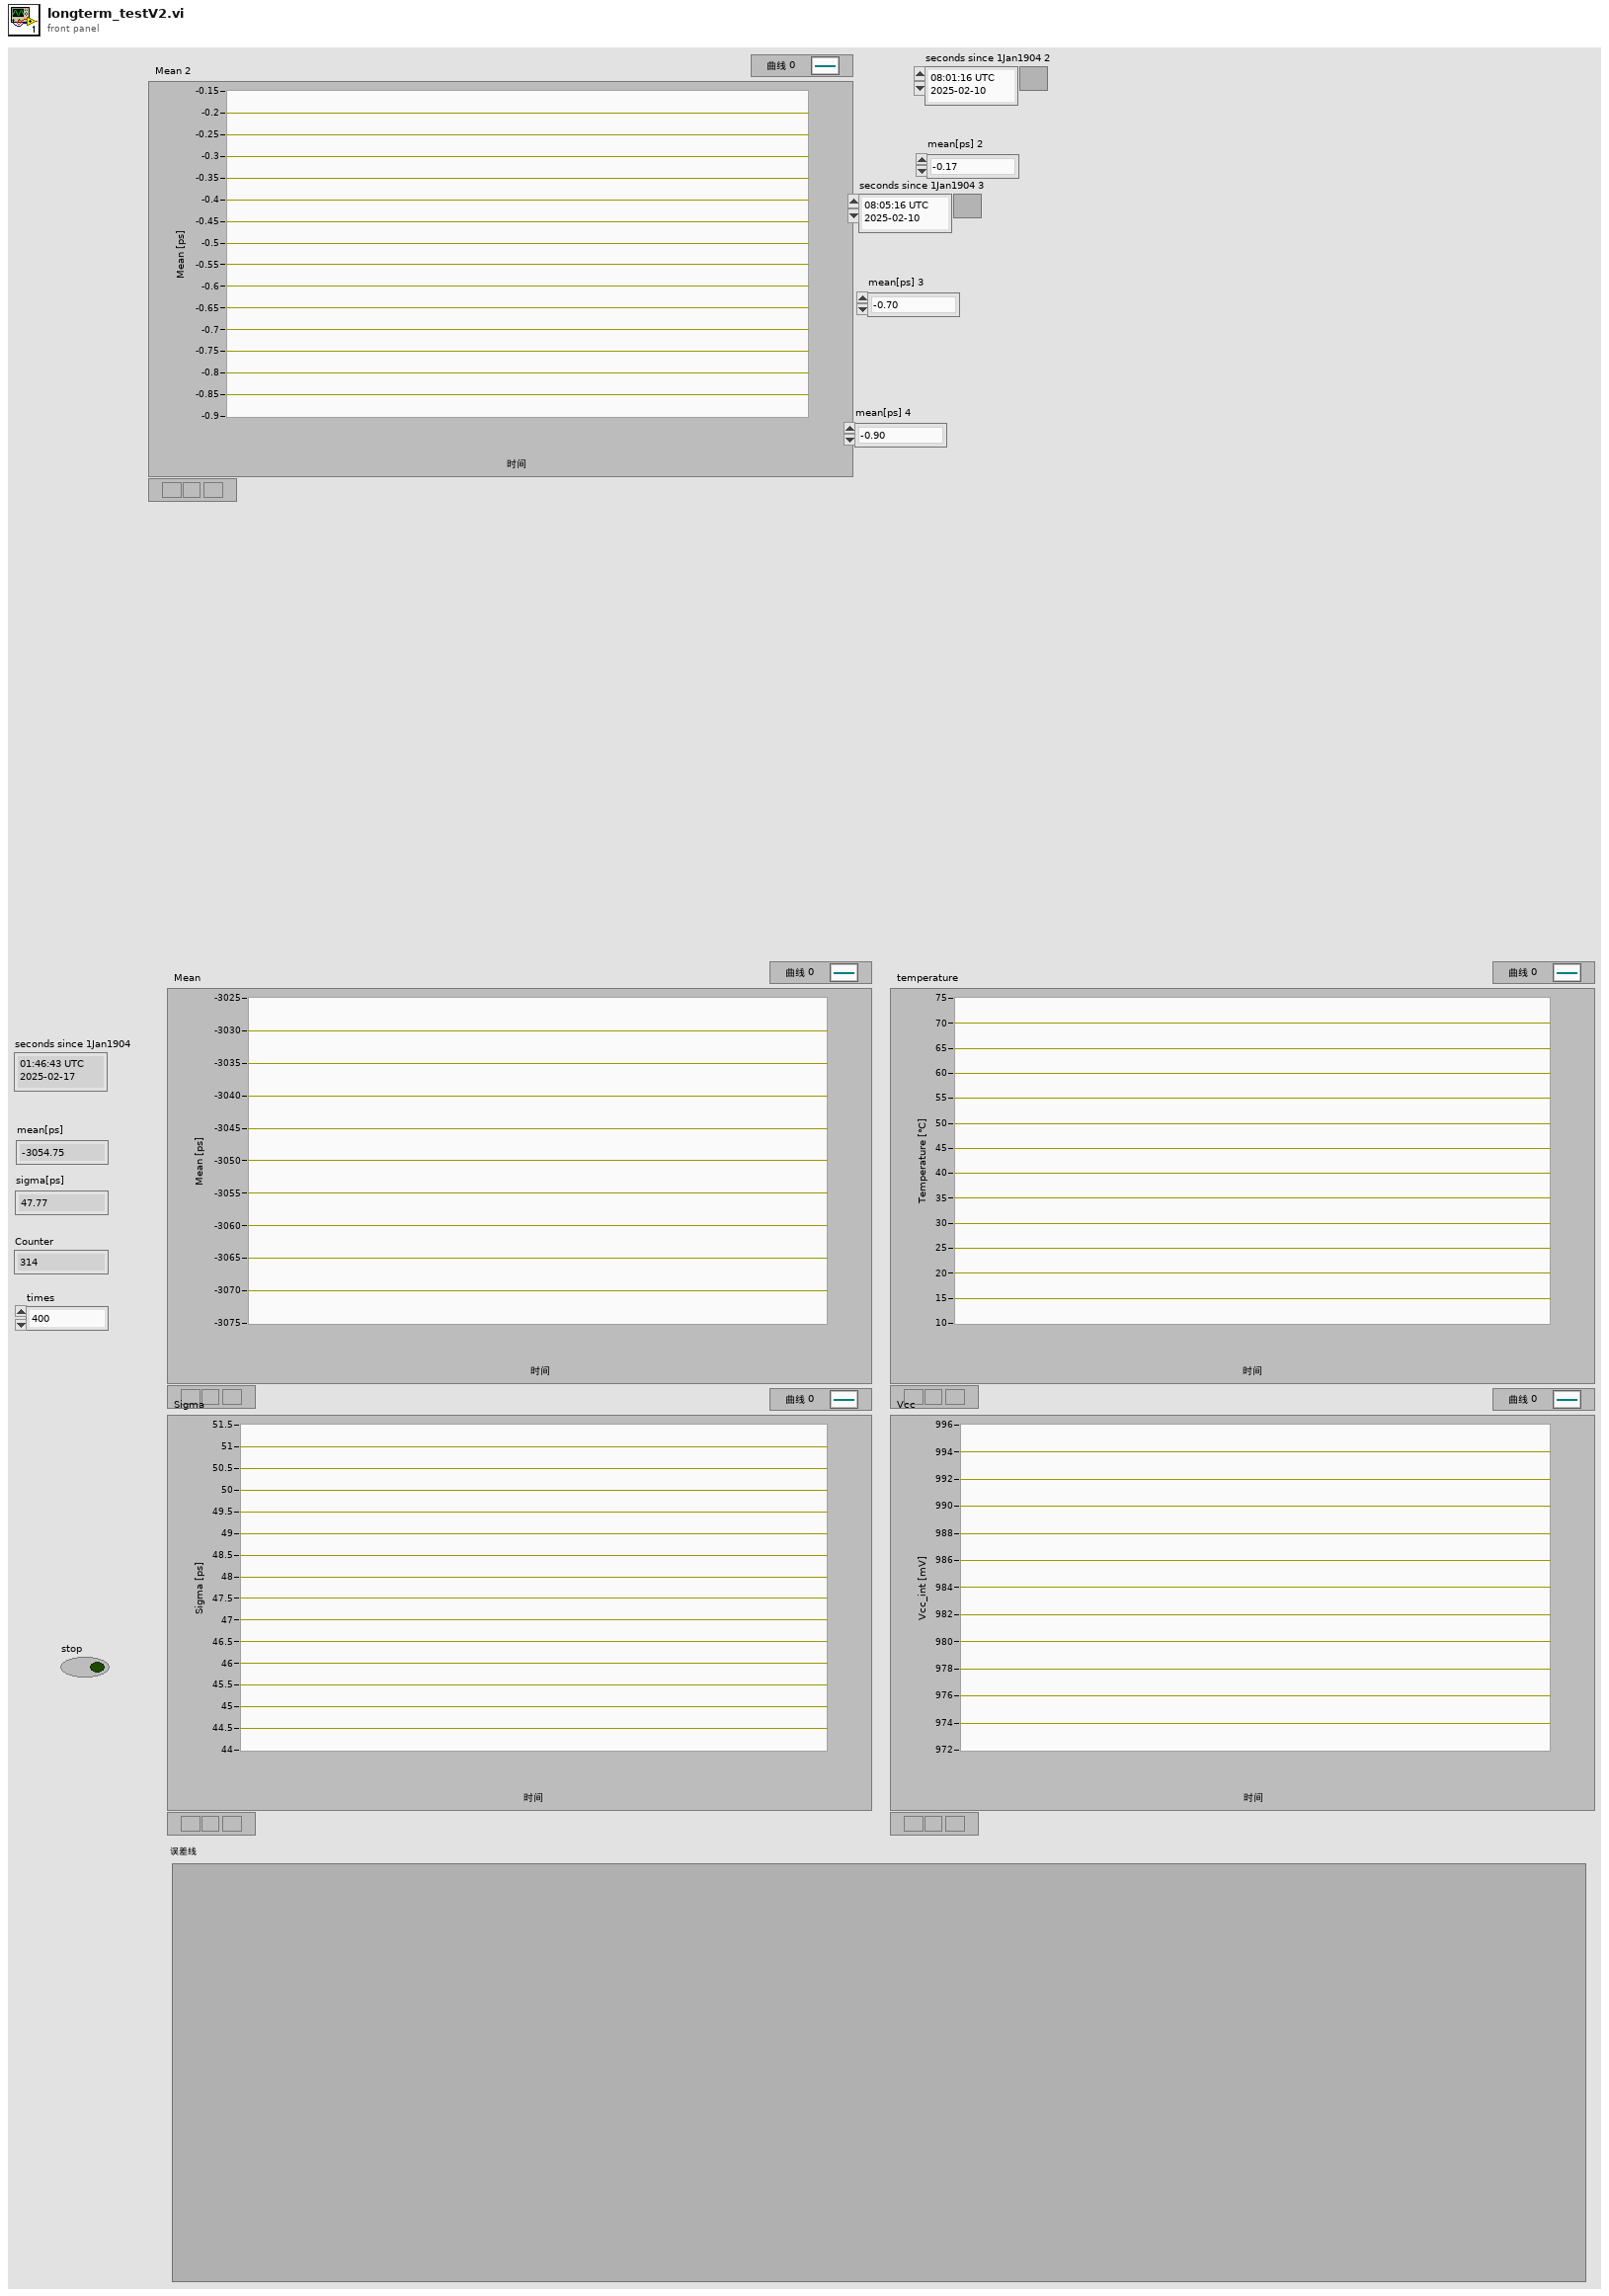
[diagram p1: front panel]
types:
  T1 = cluster{"seconds since 1Jan1904":timestamp, "mean[ps]":dbl}[]
  T2 = cluster{cluster{"seconds since 1Jan1904 2":timestamp, "mean[ps] 2":dbl}[]}[]
  T3 = cluster{"seconds since 1Jan1904":timestamp, "mean[ps]":dbl}
  T4 = cluster{"seconds since 1Jan1904":timestamp, "Fitting Sigma":dbl}
  T5 = cluster{"seconds since 1Jan1904":timestamp, "Tc[℃]":dbl}
  T6 = cluster{"seconds since 1Jan1904":timestamp, "Vcc_int[mV]":dbl}
  T7 = cluster{"seconds since 1Jan1904":timestamp, "Fitting Sigma":dbl}[]
  T8 = cluster{"seconds since 1Jan1904":timestamp, "Tc[℃]":dbl}[]
  T9 = cluster{"seconds since 1Jan1904":timestamp, "Vcc_int[mV]":dbl}[]
  T10 = cluster{"seconds since 1Jan1904 3":timestamp, "mean[ps] 4":dbl}
  T11 = cluster{"seconds since 1Jan1904 3":timestamp, "mean[ps] 3":dbl}
  T12 = cluster{"seconds since 1Jan1904 2":timestamp, "mean[ps] 2":dbl}
  T13 = cluster{"seconds since 1Jan1904 3":timestamp, "mean[ps] 3":dbl}[]
  T14 = cluster{"seconds since 1Jan1904 3":timestamp, "mean[ps] 4":dbl}[]
  T15 = cluster{cluster{"seconds since 1Jan1904 3":timestamp, "mean[ps] 3":dbl}[]}
  T16 = cluster{cluster{"seconds since 1Jan1904 3":timestamp, "mean[ps] 4":dbl}[]}
  T17 = cluster{cluster{"seconds since 1Jan1904 3":timestamp, "mean[ps] 4":dbl}[]}[]
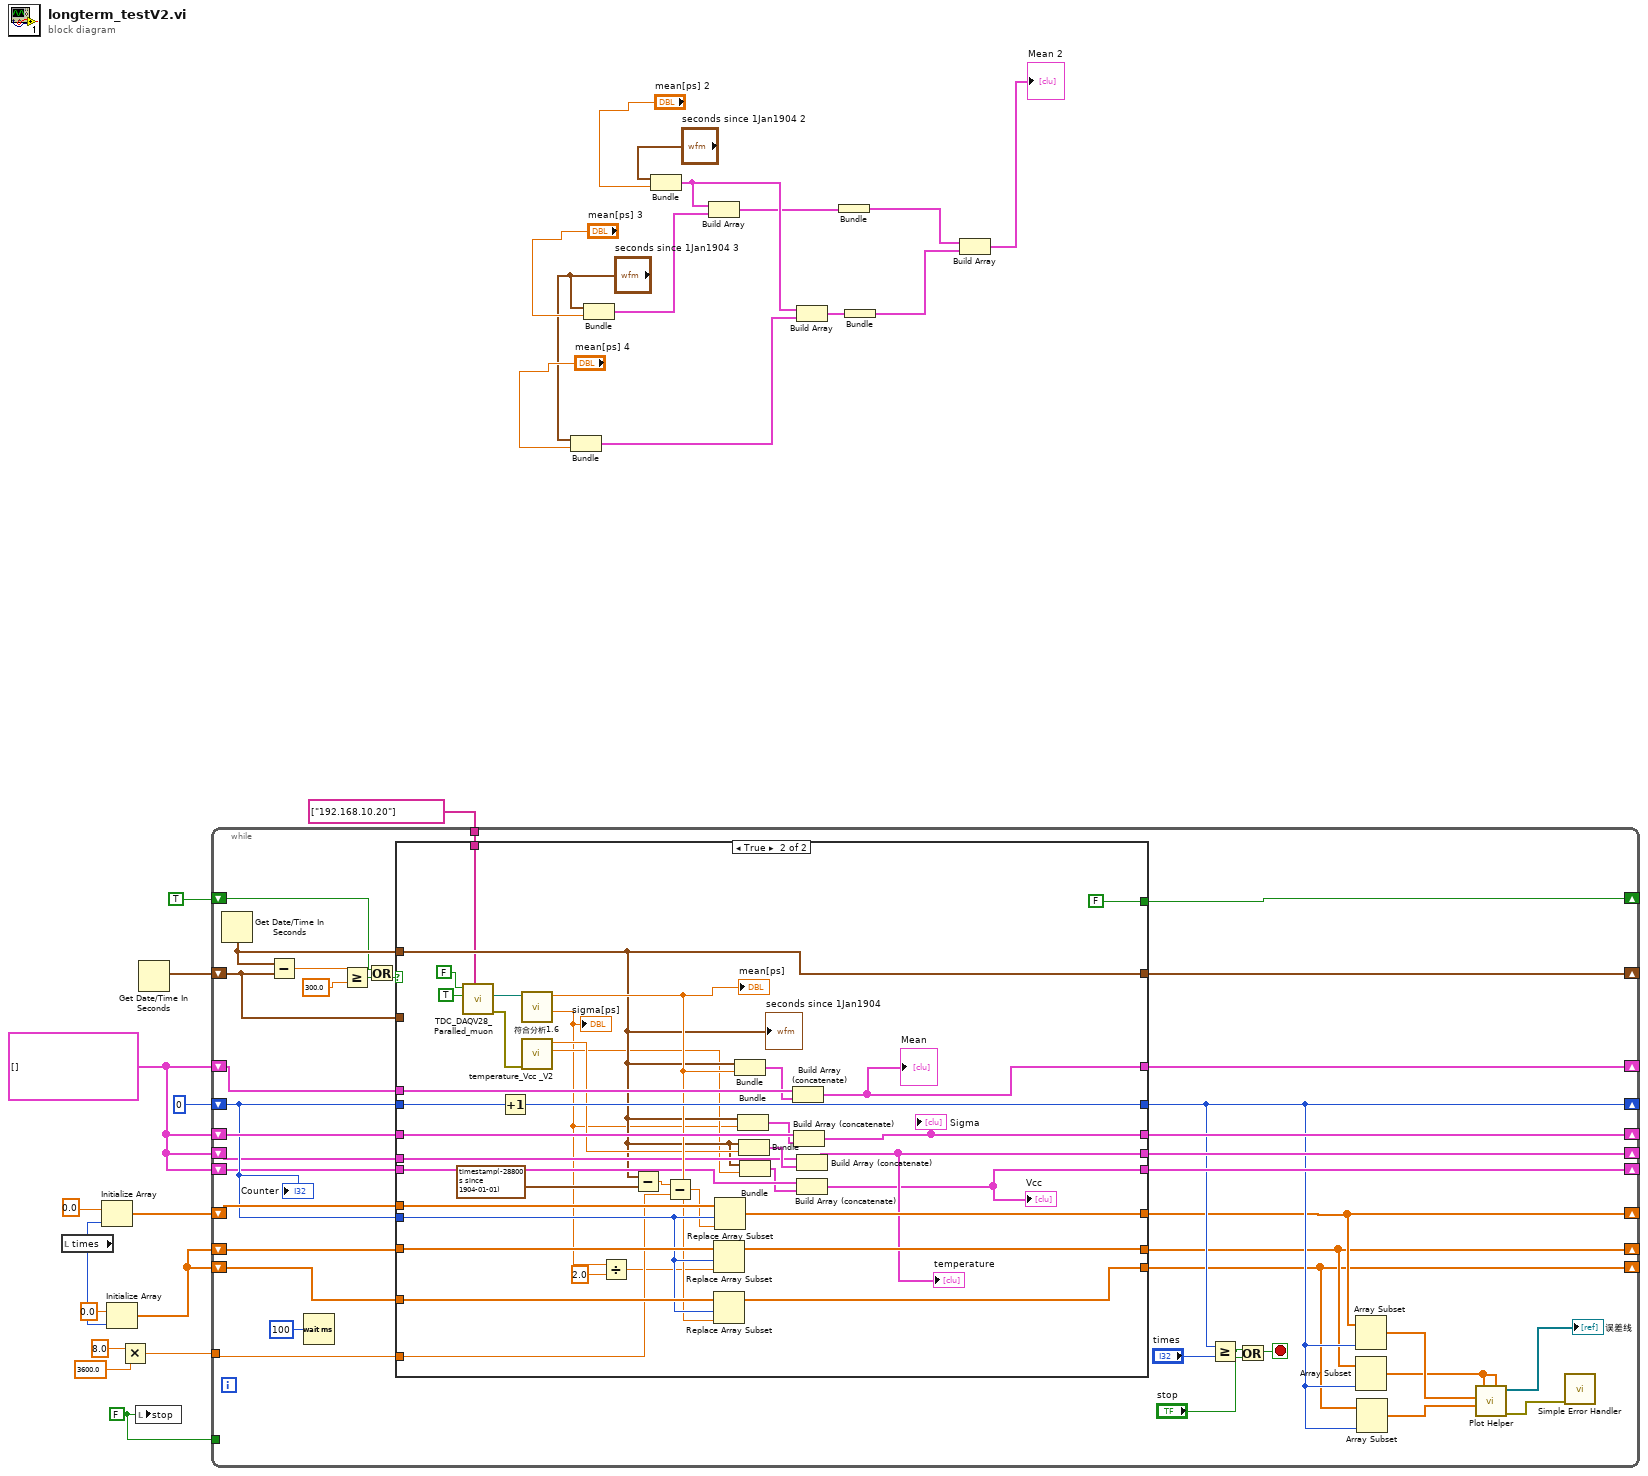
[diagram p0: block diagram]
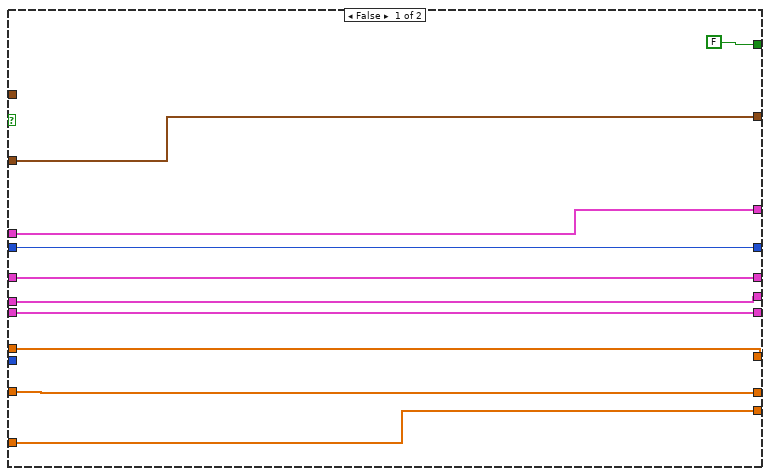
[diagram p2: hidden frame]
diagram:
  w16 = FALSE ("stop")
  w15 = T1 []
  n1 = local read "times"() -> (w23:i32)
  n2 = Initialize Array(0.0 ("mean[ps]"), w23) -> (w24:dbl[])
  n3 = Initialize Array(0.0 ("mean[ps]"), w23) -> (w22:dbl[])
  n4 = Multiply(x=8.0, y=3600.0) -> (x*y=w17:dbl)
  n5 = local write "stop"(w16) -> ()
  n6 = Get Date/Time In Seconds() -> (seconds since 1Jan1904=w27:timestamp)
  n7 = while {
    shift-right: [w60] -> _
    shift-left: w27 -> [w61]
    shift-right: [w31] -> _
    shift-left: 0 -> [w48]
    shift-right: [w54] -> _
    shift-left: TRUE -> [w55]
    shift-right: [w52] -> _
    shift-left: w15 -> [w53]
    shift-right: [w50] -> _
    shift-left: w15 -> [w51]
    shift-right: [w30] -> _
    shift-left: w24 -> [w49]
    shift-right: [w29] -> _
    shift-left: w22 -> [w47]
    shift-right: [w28] -> _
    shift-left: w22 -> [w46]
    tunnel: w17 -> [w45]
    tunnel: w16 -> [_]
    shift-right: [w40] -> _
    shift-left: w15 -> [w41]
    shift-right: [w38] -> _
    shift-left: w15 -> [w39]
    tunnel: string[] ["192.168.10.20"] ("address") -> [w37]
    stop <- w43 stop-if-true
    n8 = Get Date/Time In Seconds() -> (seconds since 1Jan1904=w59:timestamp)
    n9 = Subtract(x=w59, y=w61) -> (x-y=w64:dbl)
    n10 = Wait (ms)(milliseconds to wait=u32 100 ("等待时间（毫秒）")) -> ()  [unwired: 1 out]
    n11 = Greater Or Equal?(x=w64, y=300.0) -> (x >= y?=w62:bool)
    n12 = Or(x=w55, y=w62) -> (x .or. y?=w56:bool)
    n13 = case shown="True" w56 {
      tunnel: w61 -> [w74 _]
      tunnel: [w74 w87] -> w60
      tunnel: w59 -> [_ w87]
      tunnel: w48 -> [w73 w112]
      tunnel: [w73 w100] -> w31
      tunnel: [FALSE FALSE] -> w54
      tunnel: w53 -> [w71 w110]
      tunnel: [w71 w109] -> w52
      tunnel: w51 -> [w70 w107]
      tunnel: [w70 w105] -> w50
      tunnel: w49 -> [w69 w104]
      tunnel: w48 -> [_ w99]
      tunnel: w47 -> [w68 w102]
      tunnel: w46 -> [w67 w101]
      tunnel: [w69 w97] -> w30
      tunnel: [w68 w93] -> w29
      tunnel: [w67 w92] -> w28
      tunnel: w45 -> [_ w96]
      tunnel: w41 -> [w66 w89]
      tunnel: [w66 w82] -> w40
      tunnel: w39 -> [w65 w88]
      tunnel: [w65 w75] -> w38
      tunnel: w37 -> [_ w81]
      frame False {
      }
      frame True {
        n14 = call "TDC_DAQV28_Paralled_muon.vi"("address"=w81, "save data"=TRUE, "SMA mode"=FALSE) -> ("error out 3"=w83:errorcluster, "csv path"=w84:path)  [unwired: 6 in, 1 out]
        n15 = Increment(x=w112) -> (x+1=w100:i32)
        n16 = call "符合分析1.6.vi"("file path (dialog if empty)"=w84) -> ("Fitting Sigma"=w77:dbl, "mean[ps]"=w98:dbl)  [unwired: 6 in, 3 out]
        "mean[ps]" <- w98
        "sigma[ps]" <- w77
        n17 = call "temperature_Vcc _V2.vi"("error in (no error)"=w83) -> ("Vcc_int[mV]"=w86:dbl, "Tc[℃]"=w90:dbl)  [unwired: 8 in, 1 out]
        n18 = Divide(x=w77, y=2.0) -> (x/y=w78:dbl)
        n19 = Subtract(x=w87, y=timestamp(-28800 s since 1904-01-01) ("seconds since 1Jan1904")) -> (x-y=w95:dbl)
        n20 = Subtract(x=w95, y=w96) -> (x-y=w94:dbl)
        n21 = Replace Array Subset(array=w102, new element=w78, index=w99) -> (w93:dbl[])
        n22 = Replace Array Subset(array=w101, new element=w98, index=w99) -> (w92:dbl[])
        n23 = Replace Array Subset(array=w104, new element=w94, index=w99) -> (w97:dbl[])
        n24 = Bundle("seconds since 1Jan1904"=w87, "mean[ps]"=w98) -> (w108:T3)  [unwired: 1 in]
        n25 = Bundle("seconds since 1Jan1904"=w87, "Fitting Sigma"=w77) -> (w106:T4)  [unwired: 1 in]
        n26 = Bundle("seconds since 1Jan1904"=w87, "Tc[℃]"=w90) -> (w91:T5)  [unwired: 1 in]
        n27 = Bundle("seconds since 1Jan1904"=w87, "Vcc_int[mV]"=w86) -> (w85:T6)  [unwired: 1 in]
        n28 = Build Array (concatenate)(w110, w108) -> (w109:T1)
        "Mean" <- w109
        n29 = Build Array (concatenate)(w107, w106) -> (w105:T7)
        "Sigma" <- w105
        n30 = Build Array (concatenate)(w89, w91) -> (w82:T8)
        "temperature" <- w82
        n31 = Build Array (concatenate)(w88, w85) -> (w75:T9)
        "Vcc" <- w75
        "seconds since 1Jan1904" <- w87
      }
    }
    n32 = Greater Or Equal?(x=w31, y="times") -> (x >= y?=w44:bool)
    n33 = Or(x=w44, y="stop") -> (x .or. y?=w43:bool)
    n34 = Array Subset(array=w30, length=w31) -> (w33:dbl[])  [unwired: 1 in]
    n35 = Array Subset(array=w29, length=w31) -> (w32:dbl[])  [unwired: 1 in]
    n36 = Array Subset(array=w28, length=w31) -> (w36:dbl[])  [unwired: 1 in]
    n37 = call-poly <vilib>:"Plot Helper.vi"("error b vector"=w32, "error a vector"=w32, "y vector"=w36, "x vector"=w33) -> ("error out"=w35:errorcluster, "2D Plot Class Obj Array out"=→"误差线":refnum<class "2D Plot Datatype.lvclass">[])  [unwired: 2 in, 4 out]
    n38 = call <vilib>:"Simple Error Handler.vi"("error in (no error)"=w35) -> ()  [unwired: 4 in, 5 out]
    "Counter" <- w48
  }
  n39 = Bundle("seconds since 1Jan1904 3"="seconds since 1Jan1904 3", "mean[ps] 4"="mean[ps] 4") -> (w7:T10)  [unwired: 1 in]
  n40 = Bundle("seconds since 1Jan1904 3"="seconds since 1Jan1904 3", "mean[ps] 3"="mean[ps] 3") -> (w10:T11)  [unwired: 1 in]
  n41 = Bundle("seconds since 1Jan1904 2"="seconds since 1Jan1904 2", "mean[ps] 2"="mean[ps] 2") -> (w8:T12)  [unwired: 1 in]
  n42 = Build Array(w8, w10) -> (w6:T13)
  n43 = Build Array(w8, w7) -> (w3:T14)
  n44 = Bundle "Bundle"(w6) -> (w5:T15)  [unwired: 1 in]
  n45 = Bundle "Bundle"(w3) -> (w2:T16)  [unwired: 1 in]
  n46 = Build Array(w5, w2) -> (→"Mean 2":T17)
